vi "SR Volume.vi"() -> ()   [LabVIEW 2012]
uses:
  user.lib/SpectralRadar.llb/Data.lvclass
  user.lib/SpectralRadar.llb/Coloring.lvclass
  user.lib/SpectralRadar.llb/Colored Data.lvclass
  user.lib/SpectralRadar.llb/Colorscheme Selection.ctl
  <vilib>/Math Plots/3D Math Plots/3D Surface/3D Surface XCtrl/3D Surface.xctl
  <vilib>/Utility/error.llb/DialogType.ctl
  user.lib/SpectralRadar.llb/Coloring Byteorder.ctl
  user.lib/SpectralRadar.llb/Probe Parameter Int Selection.ctl
  user.lib/SpectralRadar.llb/Processing Parameter Int Selection.ctl
  user.lib/SpectralRadar.llb/Data Export Format Selection.ctl
  user.lib/SpectralRadar.llb/Colored Data Export Format Selection.ctl
  user.lib/SpectralRadar.llb/Normal Direction Selection.ctl
  user.lib/SpectralRadar.llb/Calibration Selection.ctl
  user.lib/SpectralRadar.llb/display Data 2D as Surface.vi
  user.lib/SpectralRadar.llb/set Scan Output.vi
  user.lib/SpectralRadar.llb/display Data 2D.vi
  user.lib/SpectralRadar.llb/OCT Device.lvclass
  user.lib/SpectralRadar.llb/LabVIEW Helper.lvlib
  user.lib/SpectralRadar.llb/Processing.lvclass
  user.lib/SpectralRadar.llb/Probe.lvclass
  user.lib/SpectralRadar.llb/Scan Pattern.lvclass
  user.lib/SpectralRadar.llb/Settings.lvclass
  user.lib/SpectralRadar.llb/Raw Data.lvclass
  user.lib/SpectralRadar.llb/Post Processing.lvlib
  user.lib/SpectralRadar.llb/ImageField.lvclass
  user.lib/SpectralRadar.llb/FullRange.lvclass
  user.lib/SpectralRadar.llb/FileSelection.lvlib
panel:
  in  "Opacity":sgl(slide) scale=0.0..1.0
  in  "Shift Y [mm]":dbl
  in  "Shift X [mm]":dbl
  out "Filtered Surface":refnum<class "Data.lvclass">
  in  "Color Scheme":T1
  in  "Options":bool
  out "Colored Data":refnum<class "Colored Data.lvclass">
  out "Coloring":refnum<class "Coloring.lvclass">
  out "Surface":refnum<class "Data.lvclass">
  out "Volume":refnum<class "Data.lvclass">
  in  "Angle [rad]":dbl
  in  "Averaging-Binning-Ratio":dbl(slide) caption="Averaging vs. Binning" min=0.0 max=1.0 step=1.0
  in  "Averaging*Binning":i32(slide)=1 caption="Quality" min=1 max=200 step=1 scale=1.0..200.0
  out "AutoSafe":bool
  out "Progress":i32(slide) max=20 scale=0.0..128.0
  in  "Tab Control":enum32{"B-Scan", "Surface"}(tab)
  in  "Boundries":cluster{sgl, sgl}(slide)={72.22738, 40.64965} scale=-20.0..150.0
  out "Frame":sgl[][](graph)
  in  "X":dbl(slide) max=2.0 scale=0.0..2.0
  in  "Y":dbl(slide) max=3.0 scale=0.0..2.0
  in  "Z":dbl(slide) max=1.600000023841858 scale=0.0..5.12 scale format="%#_2g"
  in  "Level Surface":bool
  in  "Petzval Filter":bool
  in  "Median Filter":bool
  in  "SizeFilter":i32=3 min=3 max=15 step=2
  out "3D Surface":refnum<class "3D Plot Datatype.lvclass">[](xcontrol)
  in  "Export Format":T2(ring)
  out "Image":T3(plugin-control)
  out "Reference Intensity":sgl(slide) min=0 max=1 scale=0.0..1.0
  in  "OnlineDisplay":bool
  in  "Brightness":sgl(slide)=0.49673203 caption="Sharpness" min=0 max=1 scale=0.0..1.0
  in  "Contrast":sgl(slide)=0.53594774 caption="Sharpness" min=0 max=1 scale=0.0..1.0
  in  "Saturation":sgl(slide)=0.5294118 caption="Sharpness" min=0 max=1 scale=0.0..1.0
  in  "Light":i32(slide) min=0 max=100 step=1 scale=0.0..100.0
  in  "Description":string
  in  "Test Mode":bool
  out "Test Mode Indicator":bool
  in  "Window":T4(ring)
  out "FrameRate":sgl format="%#_3g"
  out "SpacingZ":dbl
  in  "Range Y [mm]":dbl=3.5999999046325684 caption="Bereich [mm]" min=0.0 max=10.0 step=0.05000000074505806 format="%_3f"
  out "Spacing Y [µm]":dbl=40.0 min=1.0 max=500.0 step=1.0 format="%#_3g"
  in  "Number Scans Y":i32=50 min=10 max=1000 step=1
  in  "Save":bool
  in  "Recalibrate":bool
  in  "Range X [mm]":dbl=2.5999999046325684 caption="Bereich [mm]" min=0.05000000074505806 max=10.0 step=0.05000000074505806 format="%_3f"
  out "Spacing X [µm]":dbl=2.0 min=1.0 max=500.0 step=1.0 format="%#_3g"
  in  "Number Scans X":i32=500 min=100 max=2000 step=1
  in  "Measure":bool
  in  "QuitApp":bool
  # "Stability"
  # "SNR"
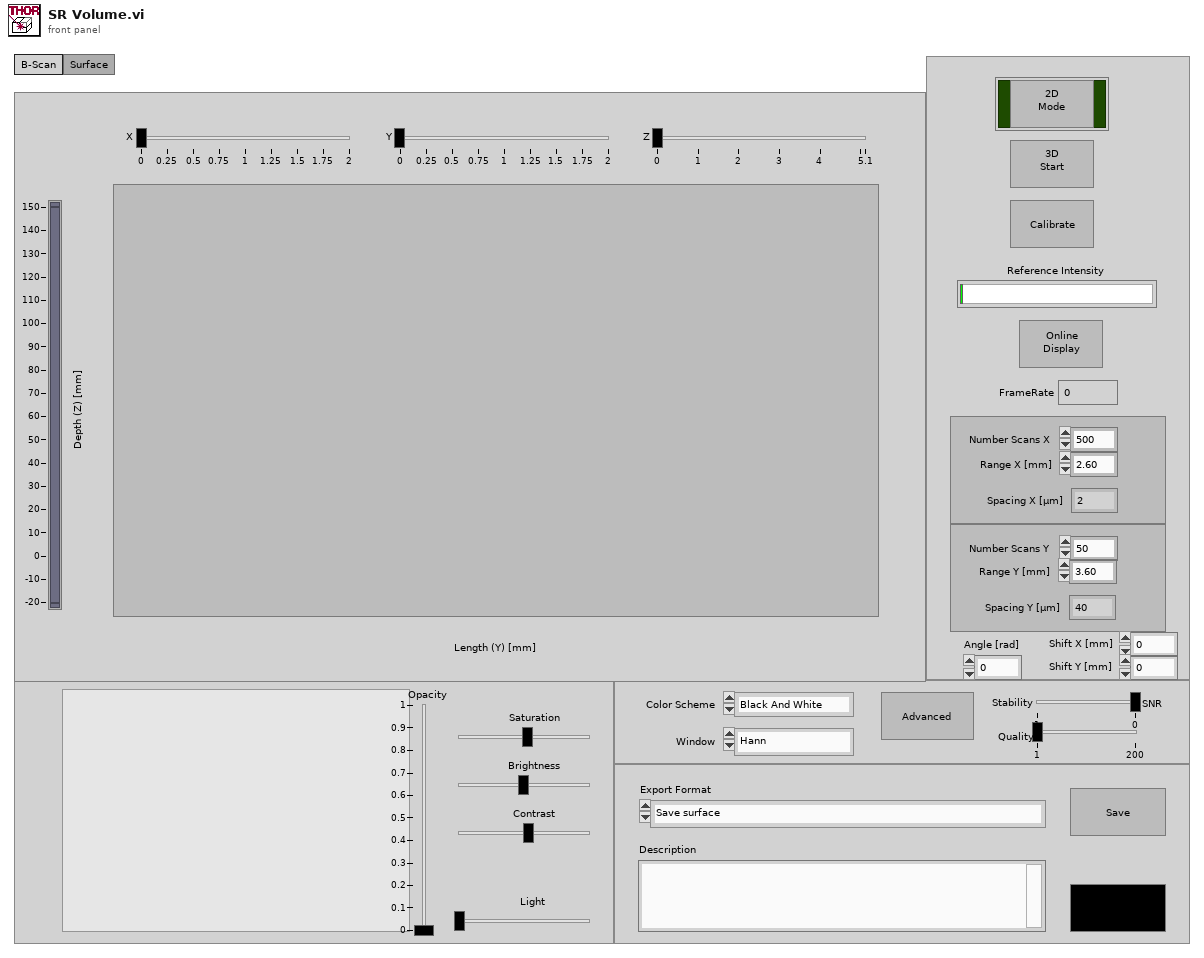
[diagram p1: front panel]
types:
  T1 = typedef "Coloring.lvclass/Colorscheme Selection.ctl" = enum16{"Black And White", "Inverted Black And White", "Color", "Black and Orange", "Black and Red", "Doppler Phase Coloring"}
  T2 = enum16{"Save surface", "Save filtered surface", "Framewise as BMP (*.bmp)", "Framewise as JPG (*.jpg)", "Framewise as PNG (*.png)", "Raw binary floating point (*.raw)", "VFF (*.vff)", "VTK (*.vtk)", "Flexible Image Transport System (*.fits)"}
  T3 = typedef "IMAQ Image.ctl" = refnum<image>
  T4 = enum16{"Hann", "Hamming", "Gauss", "Tapered Cosine", "Blackman", "4 Term B-Harris"}
  T5 = typedef "Coloring.lvclass/Coloring Byteorder.ctl" = enum16{"RGBA32", "BGRA32", "ARGB32", ""}
  T6 = enum16{"Full Well Capacity", "z Spacing", "z Range", "Dynamc Range Min [dB]", "Dynamic Range Low [dB]", "Dynamic Range High [dB]", "Dynamic Range Max [dB]"}
  T7 = typedef "Processing.lvclass/Processing Parameter Int Selection.ctl" = enum32{"Spectrum Averaging", "A-Scan Averaging", "B-Scan Averaging", "Zero Padding", "Number of Threads", "Fourier Averaging"}
  T8 = typedef "Probe.lvclass/Probe Parameter Int Selection.ctl" = enum16{"Apodization Cycles", "Oversampling", "Oversampling Slow Axis", "Speckle Reduction"}
  T9 = typedef "Data.lvclass/Data Export Format Selection.ctl" = enum16{"SRM (Spectral Radar Metafile)", "RAW", "CSV", "TXT", "Table TXT", "Fits", "VFF", "VTK", "TIFF"}
  T10 = typedef "Colored Data.lvclass/Colored Data Export Format Selection.ctl" = enum16{"SRM (Spectral Radar Metafile)", "RAW", "BMP", "PNG", "JPG", "PDF", "TIFF"}
  T11 = enum16{"Asynchronous Continuous", "Asynchronous Finite", "Synchronous"}
  T12 = typedef "Data.lvclass/Normal Direction Selection.ctl" = enum16{"Direction 1", "Direction 2", "Direction 3"}
  T13 = enum8{"Enabled", "Disabled", "Disabled and Grayed Out"}
  T14 = typedef "Processing.lvclass/Calibration Selection.ctl" = enum16{"Offset Errors", "Apodization Spectrum", "Apodization Vector", "Dispersion", "Chirp", "Extended Adjust", "Fixed Pattern"}
  T15 = typedef "DialogType.ctl" = u16
  T16 = typedef "Image Type" = u32
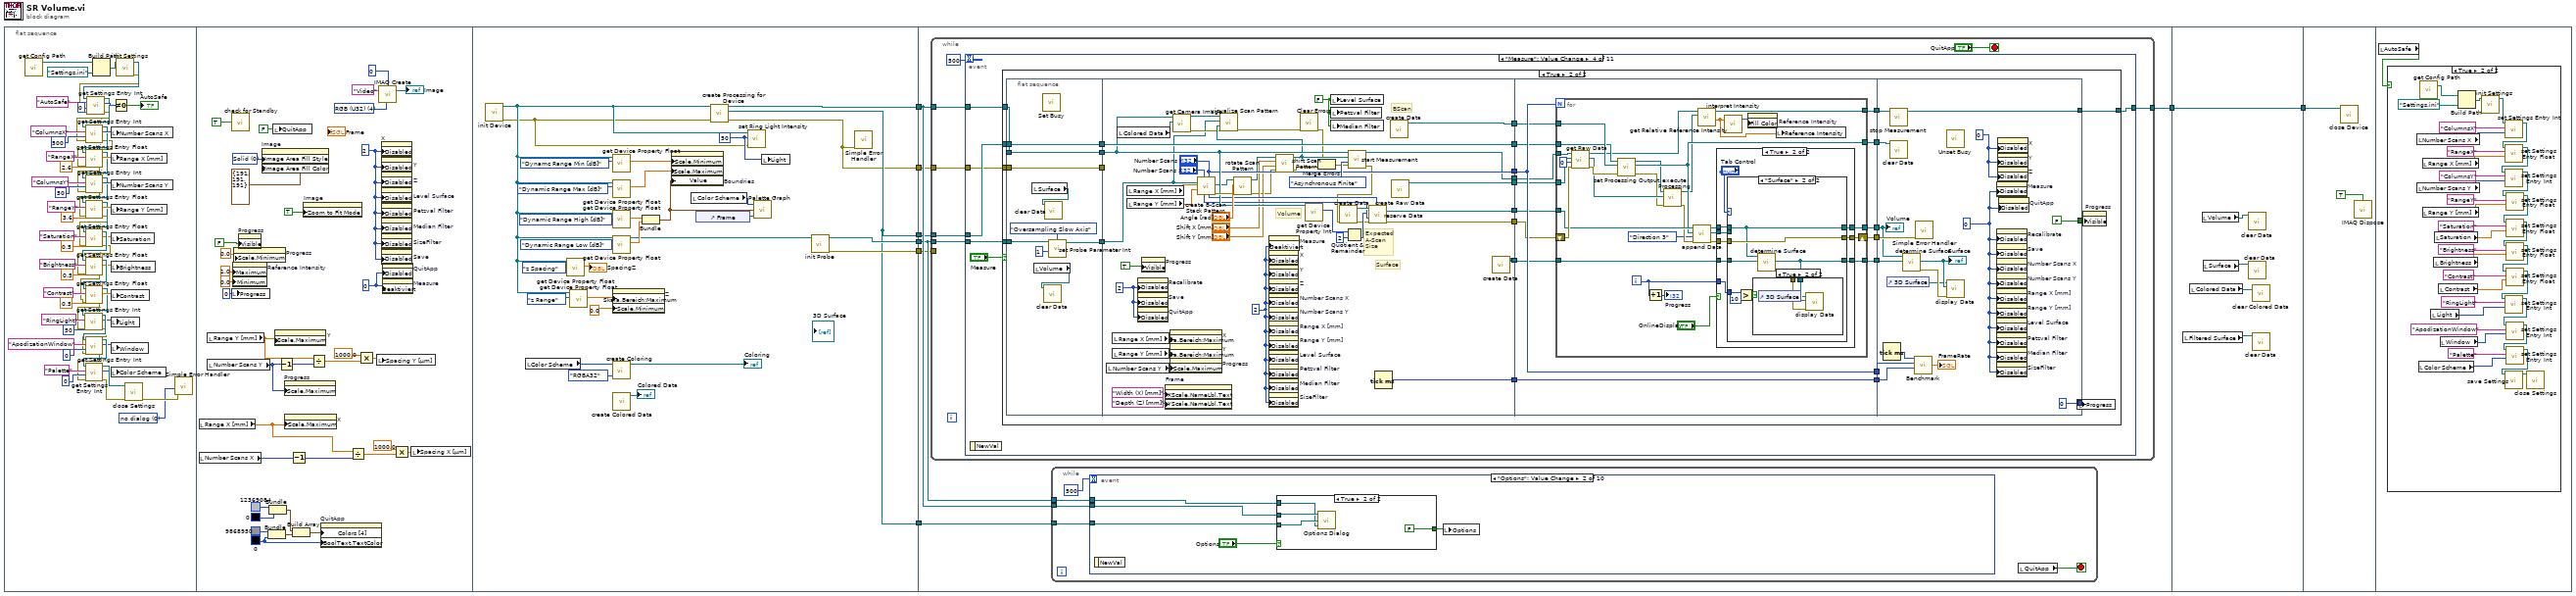
[diagram p0: block diagram]
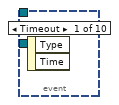
[diagram p2: hidden frame]
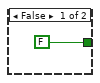
[diagram p3: hidden frame]
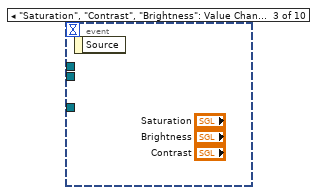
[diagram p4: hidden frame]
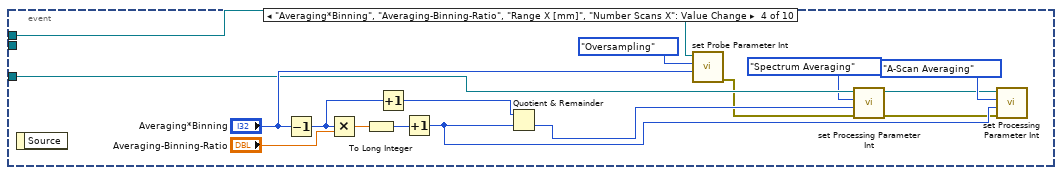
[diagram p5: hidden frame]
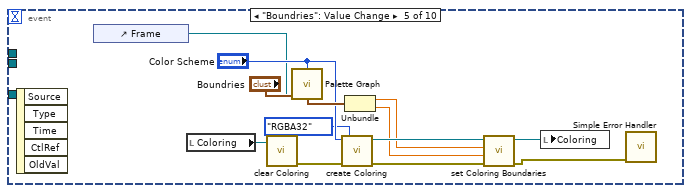
[diagram p6: hidden frame]
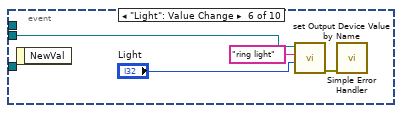
[diagram p7: hidden frame]
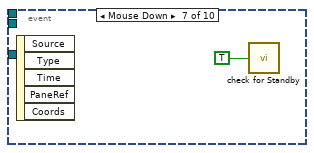
[diagram p8: hidden frame]
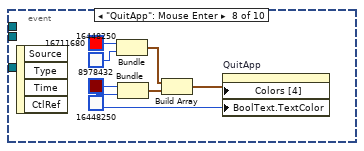
[diagram p9: hidden frame]
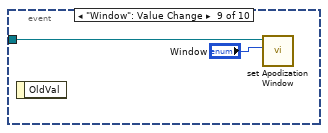
[diagram p10: hidden frame]
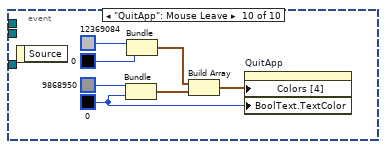
[diagram p11: hidden frame]
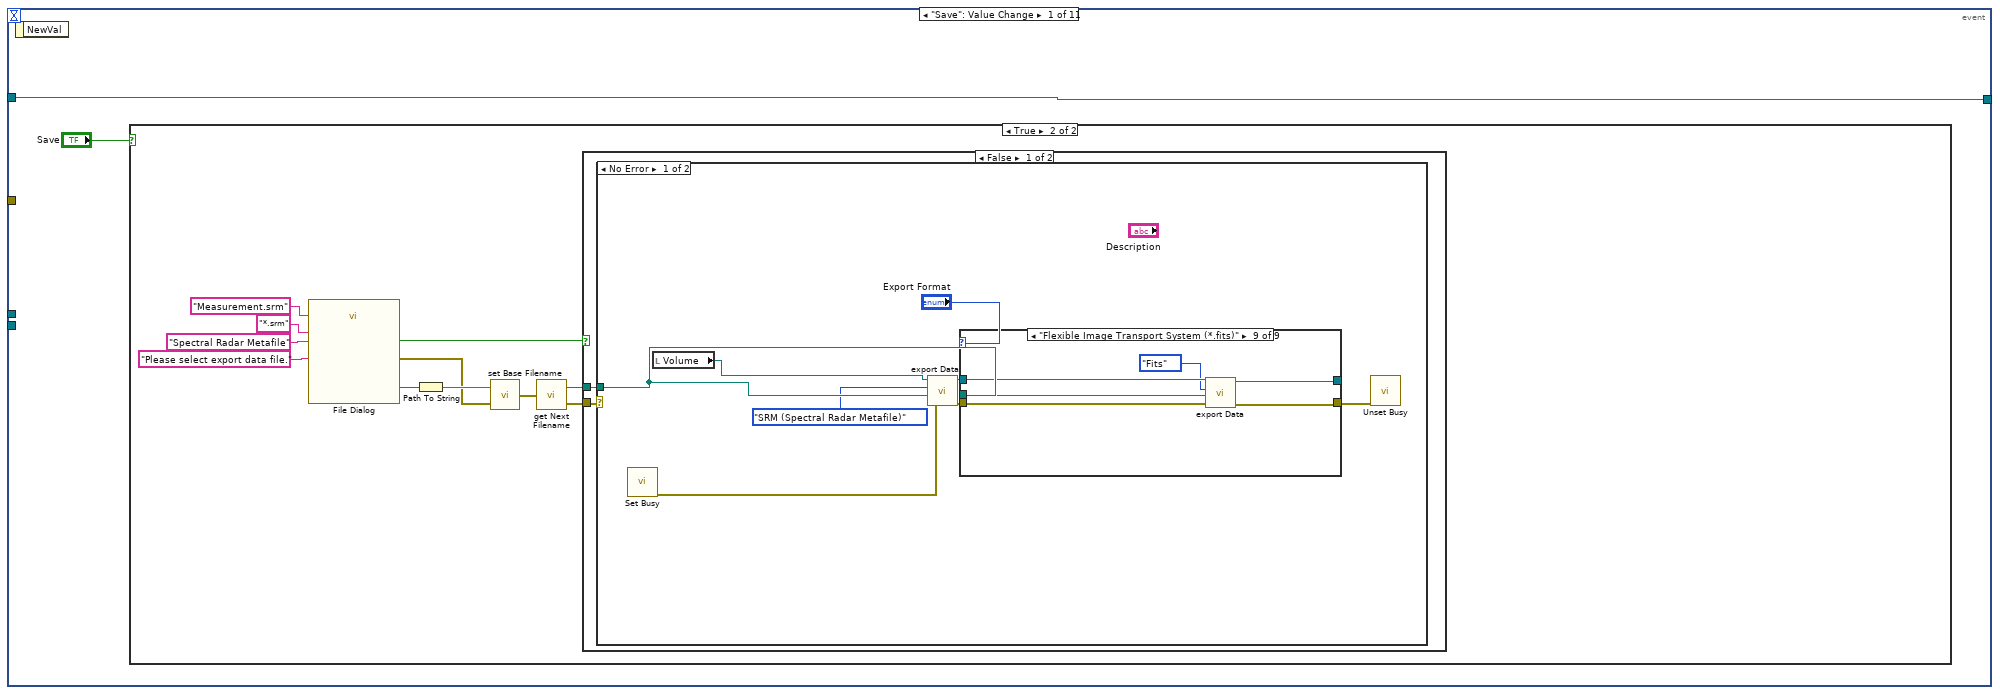
[diagram p12: hidden frame]
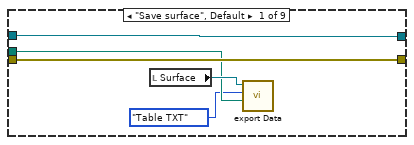
[diagram p14: hidden frame]
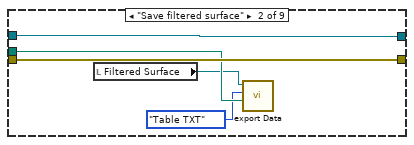
[diagram p15: hidden frame]
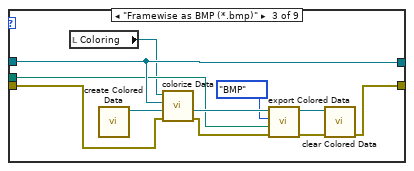
[diagram p16: hidden frame]
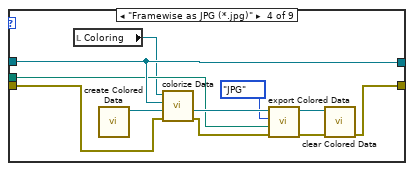
[diagram p17: hidden frame]
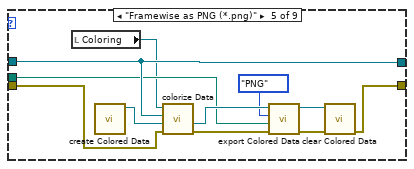
[diagram p18: hidden frame]
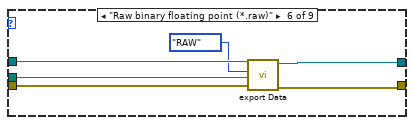
[diagram p19: hidden frame]
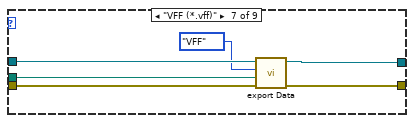
[diagram p20: hidden frame]
diagram:
  n1 = flat-sequence {
    tunnel: [w118] -> w8
    tunnel: [w119] -> w5
    tunnel: [w132] -> w4
    tunnel: [w119] -> w3
    tunnel: [w117] -> w2
    tunnel: [w130] -> w1
    tunnel: w8 -> [w141]
    tunnel: [w142] -> w6
    tunnel: w5 -> [w140]
    tunnel: w4 -> [w138]
    tunnel: w3 -> [w139]
    tunnel: w2 -> [w137]
    tunnel: w1 -> [w136]
    tunnel: [w719] -> w7
    tunnel: w6 -> [w719]
    tunnel: w7 -> [w721]
    frame #0 {
      w12 = T15 0 items=["no dialog", "OK message", "continue or stop message", "OK message + warnings", "continue/stop + warnings"] ("type of dialog (OK msg:1)")
      n2 = call "get Config Path.vi"() -> ("Path"=w22:path)  [unwired: 1 in, 1 out]
      n3 = Build Path(base path=w22, name or relative path=path "Settings.ini" ("Relative \"SpectralRadar.ini\" Path")) -> (appended path=w62:path)
      n4 = call "init Settings.vi"("Path to settings file"=w62) -> ("error out"=w9:errorcluster, "Settings"=w32:refnum<class "Settings.lvclass">)  [unwired: 5 in]
      n5 = call "get Settings Entry Int.vi"("error in (no error)"=w9, "Default Value"=0, "Node Name"="AutoSafe", "Settings"=w32) -> ("error out"=w25:errorcluster, "Value"=w35:i32, "Settings"=w31:refnum<class "Settings.lvclass">)  [unwired: 1 in]
      n6 = call "get Settings Entry Int.vi"("error in (no error)"=w25, "Default Value"=500, "Node Name"="ColumnsX", "Settings"=w31) -> ("error out"=w24:errorcluster, "Value"=w61:i32, "Settings"=w47:refnum<class "Settings.lvclass">)  [unwired: 1 in]
      n7 = call "get Settings Entry Float.vi"("error in (no error)"=w24, "Default Value"=2.6, "Node Name"="RangeX", "Settings"=w47) -> ("error out"=w23:errorcluster, "Value"=w60:dbl, "Settings"=w46:refnum<class "Settings.lvclass">)  [unwired: 1 in]
      n8 = call "get Settings Entry Int.vi"("error in (no error)"=w23, "Default Value"=50, "Node Name"="ColumnsY", "Settings"=w46) -> ("error out"=w21:errorcluster, "Value"=w59:i32, "Settings"=w45:refnum<class "Settings.lvclass">)  [unwired: 1 in]
      n9 = call "get Settings Entry Float.vi"("error in (no error)"=w21, "Default Value"=3.6, "Node Name"="RangeY", "Settings"=w45) -> ("error out"=w20:errorcluster, "Value"=w58:dbl, "Settings"=w44:refnum<class "Settings.lvclass">)  [unwired: 1 in]
      n10 = call "get Settings Entry Float.vi"("error in (no error)"=w20, "Default Value"=0.5, "Node Name"="Saturation", "Settings"=w44) -> ("error out"=w19:errorcluster, "Value"=w37:dbl, "Settings"=w43:refnum<class "Settings.lvclass">)  [unwired: 1 in]
      n11 = call "get Settings Entry Float.vi"("error in (no error)"=w19, "Default Value"=0.5, "Node Name"="Brightness", "Settings"=w43) -> ("error out"=w18:errorcluster, "Value"=w38:dbl, "Settings"=w42:refnum<class "Settings.lvclass">)  [unwired: 1 in]
      n12 = call "get Settings Entry Float.vi"("error in (no error)"=w18, "Default Value"=0.5, "Node Name"="Contrast", "Settings"=w42) -> ("error out"=w17:errorcluster, "Value"=w39:dbl, "Settings"=w30:refnum<class "Settings.lvclass">)  [unwired: 1 in]
      n13 = call "get Settings Entry Int.vi"("error in (no error)"=w17, "Default Value"=50, "Node Name"="RingLight", "Settings"=w30) -> ("error out"=w16:errorcluster, "Value"=w26:i32, "Settings"=w28:refnum<class "Settings.lvclass">)  [unwired: 1 in]
      n14 = call "get Settings Entry Int.vi"("error in (no error)"=w16, "Default Value"=0, "Node Name"="ApodizationWindow", "Settings"=w28) -> ("error out"=w15:errorcluster, "Value"=w40:i32, "Settings"=w41:refnum<class "Settings.lvclass">)  [unwired: 1 in]
      n15 = call "get Settings Entry Int.vi"("error in (no error)"=w15, "Default Value"=0, "Node Name"="Palette", "Settings"=w41) -> ("error out"=w14:errorcluster, "Value"=w11:i32, "Settings"=w36:refnum<class "Settings.lvclass">)  [unwired: 1 in]
      n16 = local write "Number Scans X"(w61) -> ()
      n17 = local write "Range X [mm]"(w60) -> ()
      n18 = local write "Number Scans Y"(w59) -> ()
      n19 = local write "Range Y [mm]"(w58) -> ()
      n20 = local write "Saturation"(w37) -> ()
      n21 = local write "Brightness"(w38) -> ()
      n22 = local write "Contrast"(w39) -> ()
      n23 = local write "Light"(w26) -> ()
      n24 = local write "Window"(w40) -> ()
      n25 = local write "Color Scheme"(w11) -> ()
      n26 = Not Equal To 0?(x=w35) -> (x != 0?=→"AutoSafe":bool)
      n27 = call "close Settings.vi"("error in (no error)"=w14, "Settings"=w36) -> ("error out"=w13:errorcluster)  [unwired: 5 in]
      n28 = call <vilib>:"Simple Error Handler.vi"("type of dialog (OK msg:1)"=w12, "error in (no error)"=w13) -> ()  [unwired: 3 in, 5 out]
    }
    frame #1 {
      w73 = T16 4 items=["Grayscale (U8)", "Grayscale (I16)", "Grayscale (SGL)", "Complex (CSG)", "RGB (U32)", "HSL (U32)", "RGB (U64)", "Grayscale (U16)"] ("Image Type")
      w77 = u8 0 ("Deaktiviert")
      w90 = u8 2 ("Disabled")
      w98 = u32 0
      w103 = u32 0 items=["Default"=3, "Solid"=0, "Hatch"=2] ("Image Area:Background:Fill Style")
      n29 = local read "Range X [mm]"() -> (w78:dbl)
      n30 = local read "Number Scans X"() -> (w80:i32)
      n31 = local read "Range Y [mm]"() -> (w85:dbl)
      n32 = local read "Number Scans Y"() -> (w86:i32)
      n33 = call "check for Standby.vi"("ResetTimer"=TRUE) -> ()  [unwired: 2 out]
      n34 = local write "Progress"(0 ("Progress")) -> ()
      n35 = property on="Reference Intensity" class="Slide (strict)"("Maximum"=1.0 ("Data Entry Limits:Maximum"), "Minimum"=0.0 ("Data Entry Limits:Minimum")) -> ()  [unwired: 2 in, 2 out]
      n36 = property on="Progress" class="Slide (strict)"("Scale.Minimum"=0.0 ("Skalieren.Bereich:Minimum")) -> ()  [unwired: 2 in, 2 out]
      n37 = property on="Progress" class="Slide (strict)"("Visible"=FALSE ("Sichtbar")) -> ()  [unwired: 2 in, 2 out]
      n38 = property on="Image" class="ImageControl"("Image Area Fill Style"=w103, "Image Area Fill Color"=cluster{"Red":u8, "Green":u8, "Blue":u8} {"Red"=191, "Green"=191, "Blue"=191} ("Image Area:Background:Fill Color")) -> ()  [unwired: 2 in, 2 out]
      n39 = Bundle(u32 9868950, w98) -> (w96:cluster{u32, u32})  [unwired: 1 in]
      n40 = Bundle(u32 12369084, u32 0) -> (w95:cluster{u32, u32})  [unwired: 1 in]
      n41 = local write "QuitApp"(FALSE ("QuitApp")) -> ()
      n42 = property on="Y" class="Slide (strict)"("Scale.Maximum"=w85) -> ()  [unwired: 2 in, 2 out]
      n43 = Decrement(x=w86) -> (x-1=w84:i32)
      n44 = property on="Progress" class="Slide (strict)"("Scale.Maximum"=w86) -> ()  [unwired: 2 in, 2 out]
      n45 = property on="X" class="Slide (strict)"("Scale.Maximum"=w78) -> ()  [unwired: 2 in, 2 out]
      n46 = Decrement(x=w80) -> (x-1=w79:i32)
      n47 = Build Array(w95, w96) -> (w97:cluster{u32, u32}[])
      n48 = property on="Image" class="ImageControl"("Zoom to Fit Mode"=TRUE) -> ()  [unwired: 2 in, 2 out]
      n49 = Divide(x=w85, y=w84) -> (x/y=w88:dbl)
      n50 = property on="QuitApp" class="Bool (strict)"("Colors [4]"=w97, "BoolText.TextColor"=w98) -> ()  [unwired: 2 in, 2 out]
      n51 = Divide(x=w78, y=w79) -> (x/y=w82:dbl)
      n52 = Multiply(x=1000.0, y=w88) -> (x*y=w89:dbl)
      n53 = local write "Spacing Y [µm]"(w89) -> ()
      n54 = call "IMAQ Create"("Border Size"=0, "Image Name"="Video", "Image Type"=w73) -> ("New Image"=→"Image":T3)  [unwired: 2 in, 1 out]
      n55 = property on="X" class="Slide (strict)"("Disabled"=w90) -> ()  [unwired: 2 in, 2 out]
      n56 = property on="Y" class="Slide (strict)"("Disabled"=w90) -> ()  [unwired: 2 in, 2 out]
      n57 = property on="Z" class="Slide (strict)"("Disabled"=w90) -> ()  [unwired: 2 in, 2 out]
      n58 = property on="Level Surface" class="Bool (strict)"("Disabled"=w90) -> ()  [unwired: 2 in, 2 out]
      n59 = property on="Petzval Filter" class="Bool (strict)"("Disabled"=w90) -> ()  [unwired: 2 in, 2 out]
      n60 = property on="Median Filter" class="Bool (strict)"("Disabled"=w90) -> ()  [unwired: 2 in, 2 out]
      n61 = property on="SizeFilter" class="DigNum (strict)"("Disabled"=w90) -> ()  [unwired: 2 in, 2 out]
      n62 = property on="Save" class="Bool"("Disabled"=w90) -> ()  [unwired: 2 in, 2 out]
      n63 = property on="QuitApp" class="Bool (strict)"("Disabled"=w77) -> ()  [unwired: 2 in, 2 out]
      n64 = property on="Measure" class="Bool"("Deaktiviert"=w77) -> ()  [unwired: 2 in, 2 out]
      n65 = Multiply(x=sgl 1000.0, y=w82) -> (x*y=w83:dbl)
      n66 = local write "Spacing X [µm]"(w83) -> ()
    }
    frame #2 {
      w135 = 50 ("Intensity[%]")
      n67 = call "init Device.vi"() -> ("error out"=w110:errorcluster, "OCTDevice"=w111:refnum<class "OCT Device.lvclass">)  [unwired: 6 in]
      n68 = local read "Color Scheme"() -> (w108:T1)
      n69 = call "get Device Property Float.vi"("Device Property Float Selection"=T6."z Spacing", "OCTDevice"=w111) -> ("Value"=→"SpacingZ":dbl)  [unwired: 3 in, 2 out]
      n70 = call "get Device Property Float.vi"("Device Property Float Selection"=T6."z Range", "OCTDevice"=w111) -> ("Value"=w115:dbl)  [unwired: 3 in, 2 out]
      n71 = call "get Device Property Float.vi"("Device Property Float Selection"=T6."Dynamc Range Min [dB]", "OCTDevice"=w111) -> ("Value"=w126:dbl)  [unwired: 3 in, 2 out]
      n72 = call "get Device Property Float.vi"("Device Property Float Selection"=T6."Dynamic Range Max [dB]", "OCTDevice"=w111) -> ("Value"=w125:dbl)  [unwired: 3 in, 2 out]
      n73 = call "get Device Property Float.vi"("Device Property Float Selection"=T6."Dynamic Range High [dB]", "OCTDevice"=w111) -> ("Value"=w121:dbl)  [unwired: 3 in, 2 out]
      n74 = call "get Device Property Float.vi"("Device Property Float Selection"=T6."Dynamic Range Low [dB]", "OCTDevice"=w111) -> ("Value"=w120:dbl, "OCTDevice"=w112:refnum<class "OCT Device.lvclass">)  [unwired: 3 in, 1 out]
      n75 = call "create Coloring.vi"("Color Byte Order"=Coloring_Byteorder."RGBA32", "Color Table Selection"=w108) -> ("Coloring"=→"Coloring":refnum<class "Coloring.lvclass">)  [unwired: 4 in, 1 out]
      n76 = property on="Z" class="Slide (strict)"("Skala.Bereich:Maximum"=w115, "Scale.Minimum"=0.0 ("Scale.Range:Minimum")) -> ()  [unwired: 2 in, 2 out]
      n77 = call "create Colored Data.vi"() -> ("Colored Data"=→"Colored Data":refnum<class "Colored Data.lvclass">)  [unwired: 6 in, 1 out]
      n78 = Bundle("Value"=w121, "Value"=w120) -> (w133:cluster{"Value":dbl, "Value":dbl})  [unwired: 1 in]
      n79 = property on="Boundries" class="Slide (strict)"("Scale.Minimum"=w126, "Scale.Maximum"=w125, "Value"=w133) -> ()  [unwired: 2 in, 2 out]
      n80 = local read "Color Scheme"() -> (w109:T1)
      n81 = control-ref of="Frame"() -> (w134:refnum<vi>)
      n82 = call "create Processing for Device.vi"("error in (no error)"=w110, "OCTDevice"=w111) -> ("error out"=w117:errorcluster, "Processing"=w119:refnum<class "Processing.lvclass">, "OCTDevice"=w118:refnum<class "OCT Device.lvclass">)  [unwired: 3 in]
      n83 = call "set Ring Light Intensity.vi"("error in (no error)"=w110, "Intensity[%]"=w135, "OCTDevice"=w111) -> ()  [unwired: 3 in, 2 out]
      n84 = call "Palette Graph.vi"("Reference to the B-scan Graph"=w134, "Boundaries"=w133, "Color Scheme"=w109) -> ()
      n85 = local write "Light"(w135) -> ()
      n86 = call "init Probe.vi"("OCT Device"=w112) -> ("error out"=w130:errorcluster, "GalvoControl"=w132:refnum<class "Probe.lvclass">)  [unwired: 5 in]
      n87 = call <vilib>:"Simple Error Handler.vi"("error in (no error)"=w117) -> ()  [unwired: 4 in, 5 out]
    }
    frame #3 {
      n88 = while {
        tunnel: w141 -> [w210]
        tunnel: [w211] -> w142
        tunnel: w140 -> [w209]
        tunnel: w138 -> [w208]
        tunnel: w137 -> [w207]
        tunnel: w136 -> [_]
        stop <- "QuitApp" stop-if-true
        n89 = event shown="[3] \"Measure\": Value Change" {
          selector: _ -> [_ _ _ _ _ _ _ _ _ _ _]
          dyn-events: _ -> [_ _ _ _ _ _ _ _ _ _ _]
          timeout: 500 -> [_ _ _ _ _ _ _ _ _ _ _]
          tunnel: w210 -> [w215 w322 w358 w366 w542 w653 w664 w670 w686 w701 w714]
          tunnel: [w215 w322 w356 w365 w540 w653 w664 w670 w686 w701 w714] -> w211
          tunnel: w209 -> [_ _ _ w362 w538 _ _ w669 _ _ _]
          tunnel: w208 -> [_ w321 _ w364 w539 _ _ _ _ _ _]
          tunnel: w207 -> [_ _ _ w361 _ _ _ _ _ _ _]
          event "Save": Value Change {
            n90 = event-data() -> ()  [unwired: 1 in, 1 out]
            n91 = case shown="True" "Save" {
              frame False {
              }
              frame True {
                n92 = call "File Dialog"("prompt"="Please select export data file.", "default name"="Measurement.srm", "pattern (all files)"="*.srm", "pattern label"="Spectral Radar Metafile") -> ("selected path"=w220:path, "cancelled"=w218:bool, "error out"=w217:errorcluster)  [unwired: 8 in, 1 out]
                n93 = Path To String(path=w220) -> (string=w219:string)
                n94 = call "set Base Filename.vi"("error in (no error)"=w217, "Base"=w219) -> ("error out"=w226:errorcluster)
                n95 = call "get Next Filename.vi"("error in (no error)"=w226) -> ("Next File Name"=w225:path, "error out"=w216:errorcluster)
                n96 = case shown="False" w218 {
                  tunnel: w225 -> [w228 _]
                  tunnel: w216 -> [w227 _]
                  frame False {
                    n97 = case shown="No Error" w227 {
                      tunnel: w228 -> [w231 _]
                      frame No Error {
                        n98 = call <vilib>:"Set Busy.vi"() -> ("error out"=w233:errorcluster)  [unwired: 10 in, 1 out]
                        n99 = local read "Volume"() -> (w229:refnum<class "Data.lvclass">)
                        n100 = call "export Data.vi"("error in (no error)"=w233, "Export File"=w231, "Data Export Format Selection"=Data_Export_Format_Selection."SRM (Spectral Radar Metafile)" ("Data 2D Export Format Selection"), "Data in"=w229) -> ("error out"=w234:errorcluster, "Data out"=w235:refnum<class "Data.lvclass">)  [unwired: 2 in]
                        n101 = case shown="\"Flexible Image Transport System (*.fits)\"" "Export Format" {
                          tunnel: w235 -> [w240 w245 w257 w268 w279 w285 w291 w296 w303]
                          tunnel: [w240 w245 w257 w268 w279 w284 w290 w297 w302] -> _
                          tunnel: w231 -> [w238 w244 w254 w265 w276 w280 w287 w293 w299]
                          tunnel: w234 -> [w241 w246 w251 w262 w273 w283 w289 w295 w301]
                          tunnel: [w241 w246 w248 w259 w270 w282 w288 w294 w300] -> w232
                          frame "Save surface", Default {
                            n102 = local read "Surface"() -> (w239:refnum<class "Data.lvclass">)
                            n103 = call "export Data.vi"("Export File"=w238, "Data Export Format Selection"=Data_Export_Format_Selection."Table TXT" ("Data 2D Export Format Selection"), "Data in"=w239) -> ()  [unwired: 3 in, 2 out]
                          }
                          frame "Save filtered surface" {
                            n104 = local read "Filtered Surface"() -> (w243:refnum<class "Data.lvclass">)
                            n105 = call "export Data.vi"("Export File"=w244, "Data Export Format Selection"=Data_Export_Format_Selection."Table TXT" ("Data 2D Export Format Selection"), "Data in"=w243) -> ()  [unwired: 3 in, 2 out]
                          }
                          frame "Framewise as BMP (*.bmp)" {
                            n106 = local read "Coloring"() -> (w247:refnum<class "Coloring.lvclass">)
                            n107 = call "create Colored Data.vi"() -> ("Colored Data"=w256:refnum<class "Colored Data.lvclass">)  [unwired: 6 in, 1 out]
                            n108 = call "colorize Data.vi"("error in (no error)"=w251, "Colored Data"=w256, "Data"=w257, "Coloring in"=w247) -> ("error out"=w250:errorcluster, "Colored Data"=w255:refnum<class "Colored Data.lvclass">)  [unwired: 2 out]
                            n109 = call "export Colored Data.vi"("error in (no error)"=w250, "File Name"=w254, "Colored Data Export Format Selection"=Colored_Data_Export_Format_Selection."BMP", "Colored Data in"=w255) -> ("error out"=w249:errorcluster, "Colored Data out"=w252:refnum<class "Colored Data.lvclass">)  [unwired: 2 in]
                            n110 = call "clear Colored Data.vi"("error in (no error)"=w249, "Colored Data"=w252) -> ("error out"=w248:errorcluster)  [unwired: 5 in]
                          }
                          frame "Framewise as JPG (*.jpg)" {
                            n111 = local read "Coloring"() -> (w258:refnum<class "Coloring.lvclass">)
                            n112 = call "create Colored Data.vi"() -> ("Colored Data"=w267:refnum<class "Colored Data.lvclass">)  [unwired: 6 in, 1 out]
                            n113 = call "colorize Data.vi"("error in (no error)"=w262, "Colored Data"=w267, "Data"=w268, "Coloring in"=w258) -> ("error out"=w261:errorcluster, "Colored Data"=w266:refnum<class "Colored Data.lvclass">)  [unwired: 2 out]
                            n114 = call "export Colored Data.vi"("error in (no error)"=w261, "File Name"=w265, "Colored Data Export Format Selection"=Colored_Data_Export_Format_Selection."JPG", "Colored Data in"=w266) -> ("error out"=w260:errorcluster, "Colored Data out"=w263:refnum<class "Colored Data.lvclass">)  [unwired: 2 in]
                            n115 = call "clear Colored Data.vi"("error in (no error)"=w260, "Colored Data"=w263) -> ("error out"=w259:errorcluster)  [unwired: 5 in]
                          }
                          frame "Framewise as PNG (*.png)" {
                            n116 = local read "Coloring"() -> (w269:refnum<class "Coloring.lvclass">)
                            n117 = call "create Colored Data.vi"() -> ("Colored Data"=w278:refnum<class "Colored Data.lvclass">)  [unwired: 6 in, 1 out]
                            n118 = call "colorize Data.vi"("error in (no error)"=w273, "Colored Data"=w278, "Data"=w279, "Coloring in"=w269) -> ("error out"=w272:errorcluster, "Colored Data"=w277:refnum<class "Colored Data.lvclass">)  [unwired: 2 out]
                            n119 = call "export Colored Data.vi"("error in (no error)"=w272, "File Name"=w276, "Colored Data Export Format Selection"=Colored_Data_Export_Format_Selection."PNG", "Colored Data in"=w277) -> ("error out"=w271:errorcluster, "Colored Data out"=w274:refnum<class "Colored Data.lvclass">)  [unwired: 2 in]
                            n120 = call "clear Colored Data.vi"("error in (no error)"=w271, "Colored Data"=w274) -> ("error out"=w270:errorcluster)  [unwired: 5 in]
                          }
                          frame "Raw binary floating point (*.raw)" {
                            n121 = call "export Data.vi"("error in (no error)"=w283, "Export File"=w280, "Data Export Format Selection"=Data_Export_Format_Selection."RAW" ("Data 2D Export Format Selection"), "Data in"=w285) -> ("error out"=w282:errorcluster, "Data out"=w284:refnum<class "Data.lvclass">)  [unwired: 2 in]
                          }
                          frame "VFF (*.vff)" {
                            n122 = call "export Data.vi"("error in (no error)"=w289, "Export File"=w287, "Data Export Format Selection"=Data_Export_Format_Selection."VFF" ("Data 2D Export Format Selection"), "Data in"=w291) -> ("error out"=w288:errorcluster, "Data out"=w290:refnum<class "Data.lvclass">)  [unwired: 2 in]
                          }
                          frame "VTK (*.vtk)" {
                            n123 = call "export Data.vi"("error in (no error)"=w295, "Export File"=w293, "Data Export Format Selection"=Data_Export_Format_Selection."VTK" ("Data 2D Export Format Selection"), "Data in"=w296) -> ("error out"=w294:errorcluster, "Data out"=w297:refnum<class "Data.lvclass">)  [unwired: 2 in]
                          }
                          frame "Flexible Image Transport System (*.fits)" {
                            n124 = call "export Data.vi"("error in (no error)"=w301, "Export File"=w299, "Data Export Format Selection"=Data_Export_Format_Selection."Fits" ("Data 2D Export Format Selection"), "Data in"=w303) -> ("error out"=w300:errorcluster, "Data out"=w302:refnum<class "Data.lvclass">)  [unwired: 2 in]
                          }
                        }
                        n125 = call <vilib>:"Unset Busy.vi"("error in (no error)"=w232) -> ()  [unwired: 10 in, 1 out]
                      }
                      frame Error {
                      }
                    }
                  }
                  frame True {
                  }
                }
              }
            }
          }
          event "Median Filter", "Level Surface", "Petzval Filter", "SizeFilter", "Spacing Y [µm]", "Spacing X [µm]": Value Change {
            n126 = event-data() -> ()  [unwired: 1 in, 1 out]
            n127 = local read "Filtered Surface"() -> (w305:refnum<class "Data.lvclass">)
            n128 = call "clear Data.vi"("Data"=w305) -> ("error out"=w306:errorcluster)  [unwired: 6 in]
            n129 = local read "Surface"() -> (w317:refnum<class "Data.lvclass">)
            n130 = call "create Data.vi"("error in (no error)"=w306) -> ("Data"=w316:refnum<class "Data.lvclass">)  [unwired: 5 in, 1 out]
            n131 = call "copy Data.vi"("Data Destination in"=w316, "Data Source in"=w317) -> ("error out"=w313:errorcluster, "Data Destination out"=w315:refnum<class "Data.lvclass">)  [unwired: 3 in, 1 out]
            n132 = case shown="True" "Median Filter" {
              tunnel: w313 -> [w344 w347]
              tunnel: w315 -> [w345 w349]
              tunnel: [w345 w348] -> w314
              tunnel: [w344 w346] -> w312
              frame False {
              }
              frame True {
                n133 = call "median Filter.vi"("error in (no error)"=w347, "Rank"="SizeFilter", "Data in"=w349) -> ("error out"=w346:errorcluster, "Data out"=w348:refnum<class "Data.lvclass">)  [unwired: 3 in]
              }
            }
            n134 = case shown="True" "Petzval Filter" {
              tunnel: w321 -> [_ _]
              tunnel: w314 -> [w330 w336]
              tunnel: w312 -> [w329 w343]
              tunnel: [w330 w335] -> w311
              tunnel: [w329 w332] -> w310
              frame False {
              }
              frame True {
                n135 = call "get Config Path.vi"() -> ("Path"=w340:path)  [unwired: 1 in, 1 out]
                n136 = call "create Image Field.vi"("error in (no error)"=w343) -> ("error out"=w341:errorcluster, "ImageField out"=w342:refnum<class "ImageField.lvclass">)  [unwired: 5 in]
                n137 = Build Path(base path=w340, name or relative path=path "ImageField.dat") -> (appended path=w337:path)
                n138 = call "load Image Field.vi"("error in (no error)"=w341, "Path"=w337, "ImageField in"=w342) -> ("error out"=w338:errorcluster, "ImageField out"=w339:refnum<class "ImageField.lvclass">)  [unwired: 3 in]
                n139 = call "correct Surface.vi"("error in (no error)"=w338, "Surface Data in"=w336, "ImageField in"=w339) -> ("error out"=w333:errorcluster, "Surface Data out"=w335:refnum<class "Data.lvclass">, "ImageField out"=w334:refnum<class "ImageField.lvclass">)  [unwired: 2 in]
                n140 = call "clear Image Field.vi"("error in (no error)"=w333, "ImageField in"=w334) -> ("error out"=w332:errorcluster)  [unwired: 5 in]
              }
            }
            n141 = case shown="True" "Level Surface" {
              tunnel: [w324 w327] -> w308
              tunnel: [w323 w328] -> w309
              tunnel: w311 -> [w324 w326]
              tunnel: w310 -> [w323 w325]
              frame False {
              }
              frame True {
                n142 = call "level Data.vi"("error in (no error)"=w325, "Data in"=w326) -> ("error out"=w328:errorcluster, "Data out"=w327:refnum<class "Data.lvclass">)  [unwired: 4 in]
              }
            }
            n143 = control-ref of="3D Surface"() -> (w304:refnum<vi>)
            n144 = call-poly "display Data.vi"("error in (no error)"=w309, "Data in"=w308, "3D Surface Refnum"=w304) -> ("Data out"=→"Filtered Surface":refnum<class "Data.lvclass">)  [unwired: 2 in, 2 out]
          }
          event Timeout {
            n145 = event-data() -> ()  [unwired: 1 in, 1 out]
            n146 = call "check for Standby.vi"() -> ("TimeOut"=w360:bool)  [unwired: 1 in, 1 out]
            n147 = call "activate Standby.vi"("StandBy"=w360, "OCTDevice"=w358) -> ("OCTDevice"=w357:refnum<class "OCT Device.lvclass">)  [unwired: 4 in, 1 out]
            n148 = local read "Colored Data"() -> (w359:refnum<class "Colored Data.lvclass">)
            n149 = call "get Camera Image.vi"("Colored Data in"=w359, "OCTDevice in"=w357) -> ("error out"=w353:errorcluster, "Colored Data out"=w354:refnum<class "Colored Data.lvclass">, "OCTDevice out"=w356:refnum<class "OCT Device.lvclass">)  [unwired: 5 in]
            n150 = local read "Image"() -> (w355:T3)
            n151 = call "update Colored Data IMAQ Image.vi"("error in (no error)"=w353, "Image in"=w355, "Colored Data"=w354) -> ("error out"=w351:errorcluster, "Image out"=w352:T3)  [unwired: 2 in, 1 out]
            n152 = local write "Image"(w352) -> ()
            n153 = call <vilib>:"Clear Errors.vi"("error in (no error)"=w351) -> ()  [unwired: 6 in, 1 out]
          }
          event "Measure": Value Change {
            n154 = event-data() -> ()  [unwired: 1 in, 1 out]
            n155 = case shown="True" "Measure" {
              tunnel: w366 -> [w367 w390]
              tunnel: [w367 w394] -> w365
              tunnel: w364 -> [_ w393]
              tunnel: w362 -> [_ w392]
              tunnel: w361 -> [_ w391]
              frame False {
              }
              frame True {
                n156 = flat-sequence {
                  tunnel: w391 -> [w401]
                  tunnel: w392 -> [w402]
                  tunnel: w393 -> [w398]
                  tunnel: w390 -> [w403]
                  tunnel: [w403] -> w389
                  tunnel: [w397] -> w388
                  tunnel: [w402] -> w387
                  tunnel: [w401] -> w386
                  tunnel: ["Number Scans Y"] -> w385
                  tunnel: [w441] -> w384
                  tunnel: [w415] -> w383
                  tunnel: [w433] -> w382
                  tunnel: [w432] -> w381
                  tunnel: [w431] -> w380
                  tunnel: [w427] -> w379
                  tunnel: [w430] -> w378
                  tunnel: w389 -> [w425]
                  tunnel: w388 -> [w404]
                  tunnel: w387 -> [w433]
                  tunnel: w386 -> [_]
                  tunnel: [w408] -> w368
                  tunnel: [w462] -> w377
                  tunnel: w385 -> [w462]
                  tunnel: [w461] -> w376
                  tunnel: [w460] -> w375
                  tunnel: w384 -> [w460]
                  tunnel: w383 -> [w458]
                  tunnel: w382 -> [w457]
                  tunnel: w381 -> [w459]
                  tunnel: w380 -> [w456]
                  tunnel: w379 -> [w455]
                  tunnel: [w454] -> w374
                  tunnel: [w453] -> w373
                  tunnel: [w452] -> w372
                  tunnel: w378 -> [w451]
                  tunnel: [w450] -> w371
                  tunnel: w368 -> [w449]
                  tunnel: w377 -> [w536]
                  tunnel: [0 ("Progress")] -> w370
                  tunnel: [FALSE ("Sichtbar")] -> w369
                  tunnel: w376 -> [w533]
                  tunnel: [w532] -> w394
                  tunnel: w375 -> [w531]
                  tunnel: w374 -> [w528]
                  tunnel: w373 -> [w527]
                  tunnel: w372 -> [w524]
                  tunnel: w371 -> [w525]
                  frame #0 {
                    n157 = local read "Surface"() -> (w400:refnum<class "Data.lvclass">)
                    n158 = local read "Volume"() -> (w399:refnum<class "Data.lvclass">)
                    n159 = call <vilib>:"Set Busy.vi"() -> ()  [unwired: 10 in, 2 out]
                    n160 = call "clear Data.vi"("Data"=w399) -> ()  [unwired: 6 in, 1 out]
                    n161 = call "clear Data.vi"("Data"=w400) -> ()  [unwired: 6 in, 1 out]
                    n162 = call "set Probe Parameter Int.vi"("Value"=1, "Probe Parameter Int"=Probe_Parameter_Int_Selection."Oversampling Slow Axis", "GalvoControl"=w398) -> ("GalvoControl"=w397:refnum<class "Probe.lvclass">)  [unwired: 3 in, 1 out]
                  }
                  frame #1 {
                    w439 = FALSE ("Level Surface")
                    w442 = u8 2 ("Deaktiviert")
                    w440 = u8 2
                    # "Expected\nA-Scan\nSize"
                    # "Surface"
                    # "Volume"
                    # "BScan"
                    n163 = local read "Number Scans Y"() -> (w447:i32)
                    n164 = local read "Range X [mm]"() -> (w446:dbl)
                    n165 = local read "Range Y [mm]"() -> (w448:dbl)
                    n166 = local read "Colored Data"() -> (w429:refnum<class "Colored Data.lvclass">)
                    n167 = local read "Range X [mm]"() -> (w438:dbl)
                    n168 = local read "Range Y [mm]"() -> (w437:dbl)
                    n169 = property on="Recalibrate" class="Bool"("Disabled"=w442) -> ()  [unwired: 2 in, 2 out]
                    n170 = property on="Save" class="Bool"("Disabled"=w442) -> ()  [unwired: 2 in, 2 out]
                    n171 = property on="QuitApp" class="Bool (strict)"("Disabled"=w442) -> ()  [unwired: 2 in, 2 out]
                    n172 = property on="Progress" class="Slide (strict)"("Visible"=TRUE ("Sichtbar")) -> ()  [unwired: 2 in, 2 out]
                    n173 = property on="Frame" class="IntGraph (strict)"("XScale.NameLbl.Text"="Width (X) [mm]" ("X Scale.Name Label.Text"), "YScale.NameLbl.Text"="Depth (Z) [mm]" ("Y Scale.Name Label.Text")) -> ()  [unwired: 2 in, 2 out]
                    n174 = property on="X" class="Slide (strict)"("Skala.Bereich:Maximum"=w446) -> ()  [unwired: 2 in, 2 out]
                    n175 = property on="Y" class="Slide (strict)"("Skala.Bereich:Maximum"=w448) -> ()  [unwired: 2 in, 2 out]
                    n176 = property on="Progress" class="Slide (strict)"("Scale.Maximum"=w447) -> ()  [unwired: 2 in, 2 out]
                    n177 = call "get Camera Image.vi"("Colored Data in"=w429, "OCTDevice in"=w425) -> ("error out"=w407:errorcluster, "OCTDevice out"=w405:refnum<class "OCT Device.lvclass">)  [unwired: 5 in, 1 out]
                    n178 = call "create B-Scan Stack Pattern.vi"("Size Y"="Number Scans Y", "Size X"="Number Scans X", "Range Y"=w437, "Range X"=w438, "Probe"=w404) -> ("error out"=w434:errorcluster, "Scan Pattern"=w417:refnum<class "Scan Pattern.lvclass">)  [unwired: 2 in, 1 out]
                    n179 = call "rotate Scan Pattern.vi"("error in (no error)"=w434, "Angle"="Angle [rad]", "ScanPattern"=w417) -> ("error out"=w413:errorcluster, "ScanPattern"=w420:refnum<class "Scan Pattern.lvclass">)  [unwired: 3 in]
                    n180 = property on="X" class="Slide (strict)"("Disabled"=w440) -> ()  [unwired: 2 in, 2 out]
                    n181 = property on="Y" class="Slide (strict)"("Disabled"=w440) -> ()  [unwired: 2 in, 2 out]
                    n182 = property on="Z" class="Slide (strict)"("Disabled"=w440) -> ()  [unwired: 2 in, 2 out]
                    n183 = property on="Number Scans X" class="DigNum (strict)"("Disabled"=w440) -> ()  [unwired: 2 in, 2 out]
                    n184 = property on="Number Scans Y" class="DigNum (strict)"("Disabled"=w440) -> ()  [unwired: 2 in, 2 out]
                    n185 = property on="Range X [mm]" class="DigNum (strict)"("Disabled"=w440) -> ()  [unwired: 2 in, 2 out]
                    n186 = property on="Range Y [mm]" class="DigNum (strict)"("Disabled"=w440) -> ()  [unwired: 2 in, 2 out]
                    n187 = property on="Level Surface" class="Bool (strict)"("Disabled"=w440) -> ()  [unwired: 2 in, 2 out]
                    n188 = property on="Petzval Filter" class="Bool (strict)"("Disabled"=w440) -> ()  [unwired: 2 in, 2 out]
                    n189 = property on="Median Filter" class="Bool (strict)"("Disabled"=w440) -> ()  [unwired: 2 in, 2 out]
                    n190 = property on="SizeFilter" class="DigNum (strict)"("Disabled"=w440) -> ()  [unwired: 2 in, 2 out]
                    n191 = property on="Measure" class="Bool"("Deaktiviert"=w440) -> ()  [unwired: 2 in, 2 out]
                    n192 = call "shift Scan Pattern.vi"("error in (no error)"=w413, "Shift Y"="Shift Y [mm]", "Shift X"="Shift X [mm]", "Scan Pattern in"=w420) -> ("error out"=w412:errorcluster, "Scan Pattern out"=w416:refnum<class "Scan Pattern.lvclass">)  [unwired: 2 in]
                    n193 = call "visualize Scan Pattern.vi"("error in (no error)"=w407, "Scan Pattern in"=w416, "Probe"=w404, "OCT Device"=w405) -> ("error out"=w406:errorcluster)  [unwired: 1 in, 3 out]
                    n194 = call <vilib>:"Clear Errors.vi"("error in (no error)"=w406) -> ("error out"=w410:errorcluster)  [unwired: 6 in]
                    n195 = call "get Device Property Int.vi"("OCTDevice"=w425) -> ("Value"=w426:i32)  [unwired: 4 in, 2 out]
                    n196 = Merge Errors(w410, w412) -> (w411:errorcluster)
                    n197 = local write "Level Surface"(w439) -> ()
                    n198 = local write "Petzval Filter"(w439) -> ()
                    n199 = local write "Median Filter"(w439) -> ()
                    n200 = Quotient & Remainder(x=w426, y=2) -> (floor(x/y)=w421:i32)  [unwired: 1 out]
                    n201 = call "start Measurement.vi"("error in (no error)"=w411, "Acquisition Type"=T11."Asynchronous Finite", "Scan Pattern"=w416, "OCTDevice"=w425) -> ("error out"=w409:errorcluster, "OCTDevice"=w415:refnum<class "OCT Device.lvclass">)  [unwired: 1 in, 1 out]
                    n202 = call "create Data.vi"("error in (no error)"=w409) -> ("error out"=w414:errorcluster, "Data"=w428:refnum<class "Data.lvclass">)  [unwired: 5 in]
                    n203 = call "reserve Data.vi"("Size 3"="Number Scans Y", "error in (no error)"=w414, "Size 2"="Number Scans X", "Size 1"=w421, "Data in"=w428) -> ("error out"=w408:errorcluster, "Data out"=w427:refnum<class "Data.lvclass">)  [unwired: 3 in]
                    n204 = Tick Count (ms)() -> (millisecond timer value=w441:u32)
                    n205 = call "create Data.vi"() -> ("Data"=w432:refnum<class "Data.lvclass">)  [unwired: 6 in, 1 out]
                    n206 = call "create Raw Data.vi"() -> ("Raw Data"=w431:refnum<class "Raw Data.lvclass">)  [unwired: 6 in, 1 out]
                    n207 = call "create Data.vi"() -> ("Data"=w430:refnum<class "Data.lvclass">)  [unwired: 6 in, 1 out]
                  }
                  frame #2 {
                    n208 = for {
                      N: w462 -> [_]
                      tunnel: [w470] -> w461
                      tunnel: w459 -> [w487]
                      tunnel: w458 -> [w488]
                      tunnel: w457 -> [w486]
                      tunnel: w456 -> [w484]
                      tunnel: w455 -> [w479]
                      tunnel: [w478] -> w453
                      tunnel: [w472] -> w452
                      tunnel: w451 -> [w466]
                      tunnel: [w465] -> w450
                      shift-right: [w482] -> w454
                      shift-left: w449 -> [w489]
                      i -> [w490]
                      n209 = call "get Raw Data.vi"("error in (no error)"=w489, "Camera Index"=0, "RawData in"=w484, "OCTDevice in"=w488) -> ("error out"=w485:errorcluster, "RawData out"=w483:refnum<class "Raw Data.lvclass">, "OCTDevice out"=w471:refnum<class "OCT Device.lvclass">)  [unwired: 1 in]
                      n210 = call-poly "set Processing Output.vi"("error in (no error)"=w485, "Data"=w487, "Processing"=w486) -> ("error out"=w480:errorcluster, "Data"=w478:refnum<class "Data.lvclass">, "Processing"=w468:refnum<class "Processing.lvclass">)  [unwired: 2 in]
                      n211 = Increment(x=w490) -> (x+1=→"Progress":i32)
                      n212 = call "execute Processing.vi"("error in (no error)"=w480, "Raw Data"=w483, "Processing"=w468) -> ("error out"=w475:errorcluster, "Processing"=w467:refnum<class "Processing.lvclass">)  [unwired: 2 in, 1 out]
                      n213 = call "append Data.vi"("error in (no error)"=w475, "Normal Direction"=Normal_Direction_Selection."Direction 3", "Data to append in"=w478, "Data in"=w479) -> ("error out"=w476:errorcluster, "Data to append out"=w477:refnum<class "Data.lvclass">, "Data out"=w473:refnum<class "Data.lvclass">)  [unwired: 1 in]
                      n214 = call "get Relative Reference Intensity.vi"("Processing"=w467, "OCTDevice"=w471) -> ("Relative Reference Intensity"=w464:dbl, "OCTDevice"=w470:refnum<class "OCT Device.lvclass">)  [unwired: 2 in, 2 out]
                      n215 = case shown="True" "OnlineDisplay" {
                        tunnel: w490 -> [_ w495]
                        tunnel: w477 -> [_ w502]
                        tunnel: w476 -> [w494 w501]
                        tunnel: [w494 w500] -> w482
                        tunnel: w473 -> [w493 w499]
                        tunnel: [w493 w498] -> w472
                        tunnel: w466 -> [w492 w497]
                        tunnel: [w492 w496] -> w465
                        frame False {
                        }
                        frame True {
                          n216 = case shown="\"Surface\"" "Tab Control" {
                            tunnel: w502 -> [w509 _]
                            tunnel: w501 -> [w507 w517]
                            tunnel: [w506 w517] -> w500
                            tunnel: w499 -> [w505 w516]
                            tunnel: [w505 w516] -> w498
                            tunnel: w497 -> [w504 w515]
                            tunnel: [w504 w514] -> w496
                            tunnel: w495 -> [_ w512]
                            frame "B-Scan", Default {
                              n217 = control-ref of="Frame"() -> (w508:refnum<vi>)
                              n218 = call-poly "display Data.vi"("error in (no error)"=w507, "Data in"=w509, "IntGraph Refnum"=w508) -> ("error out"=w506:errorcluster)  [unwired: 2 in, 2 out]
                            }
                            frame "Surface" {
                              n219 = Greater?(x=w512, y=10) -> (0:w510:bool)
                              n220 = call "determine Surface.vi"("Surface Data in"=w515, "Data in"=w516) -> ("error out"=w513:errorcluster, "Surface Data out"=w514:refnum<class "Data.lvclass">)  [unwired: 3 in, 1 out]
                              n221 = case shown="True" w510 {
                                tunnel: w514 -> [_ w520]
                                tunnel: w513 -> [_ w519]
                                frame False {
                                }
                                frame True {
                                n222 = control-ref of="3D Surface"() -> (w518:refnum<vi>)
                                n223 = call-poly "display Data.vi"("error in (no error)"=w519, "Data in"=w520, "3D Surface Refnum"=w518) -> ()  [unwired: 2 in, 3 out]
                                }
                              }
                            }
                          }
                        }
                      }
                      n224 = call "interpret Intensity.vi"("Intensity"=w464) -> ("Color"=w469:u32)  [unwired: 1 in, 1 out]
                      n225 = property on="Reference Intensity" class="Slide (strict)"("Fill Color"=w469) -> ()  [unwired: 2 in, 2 out]
                      n226 = local write "Reference Intensity"(w464) -> ()
                    }
                  }
                  frame #3 {
                    w529 = u8 0 ("Deaktiviert")
                    w526 = u8 0
                    n227 = Tick Count (ms)() -> (millisecond timer value=w530:u32)
                    n228 = control-ref of="3D Surface"() -> (w521:refnum<vi>)
                    n229 = call "stop Measurement.vi"("OCTDevice"=w533) -> ("OCTDevice"=w532:refnum<class "OCT Device.lvclass">)  [unwired: 5 in, 1 out]
                    n230 = call "clear Data.vi"("Data"=w527) -> ()  [unwired: 6 in, 1 out]
                    n231 = call "determine Surface.vi"("Surface Data in"=w525, "Data in"=w524) -> ("error out"=w522:errorcluster, "Surface Data out"=w523:refnum<class "Data.lvclass">)  [unwired: 3 in, 1 out]
                    "Surface" <- w523
                    n232 = call "Benchmark.vi"("TimeStart"=w531, "NumberOfBScans"=w536, "TimeFinish"=w530) -> ("FrameRate"=→"FrameRate":sgl)  [unwired: 1 in, 2 out]
                    n233 = call <vilib>:"Simple Error Handler.vi"("error in (no error)"=w528) -> ()  [unwired: 4 in, 5 out]
                    n234 = call <vilib>:"Unset Busy.vi"() -> ()  [unwired: 11 in, 1 out]
                    n235 = call-poly "display Data.vi"("error in (no error)"=w522, "Data in"=w523, "3D Surface Refnum"=w521) -> ()  [unwired: 2 in, 3 out]
                    n236 = property on="Measure" class="Bool"("Disabled"=w526) -> ()  [unwired: 2 in, 2 out]
                    n237 = property on="Recalibrate" class="Bool"("Disabled"=w526) -> ()  [unwired: 2 in, 2 out]
                    n238 = property on="Save" class="Bool"("Disabled"=w526) -> ()  [unwired: 2 in, 2 out]
                    n239 = property on="Number Scans X" class="DigNum (strict)"("Disabled"=w526) -> ()  [unwired: 2 in, 2 out]
                    n240 = property on="Number Scans Y" class="DigNum (strict)"("Disabled"=w526) -> ()  [unwired: 2 in, 2 out]
                    n241 = property on="Range X [mm]" class="DigNum (strict)"("Disabled"=w526) -> ()  [unwired: 2 in, 2 out]
                    n242 = property on="Range Y [mm]" class="DigNum (strict)"("Disabled"=w526) -> ()  [unwired: 2 in, 2 out]
                    n243 = property on="Level Surface" class="Bool (strict)"("Disabled"=w526) -> ()  [unwired: 2 in, 2 out]
                    n244 = property on="Petzval Filter" class="Bool (strict)"("Disabled"=w526) -> ()  [unwired: 2 in, 2 out]
                    n245 = property on="Median Filter" class="Bool (strict)"("Disabled"=w526) -> ()  [unwired: 2 in, 2 out]
                    n246 = property on="SizeFilter" class="DigNum (strict)"("Disabled"=w526) -> ()  [unwired: 2 in, 2 out]
                    n247 = property on="X" class="Slide (strict)"("Disabled"=w529) -> ()  [unwired: 2 in, 2 out]
                    n248 = property on="Y" class="Slide (strict)"("Disabled"=w529) -> ()  [unwired: 2 in, 2 out]
                    n249 = property on="Z" class="Slide (strict)"("Disabled"=w529) -> ()  [unwired: 2 in, 2 out]
                    n250 = property on="QuitApp" class="Bool (strict)"("Disabled"=w526) -> ()  [unwired: 2 in, 2 out]
                    "Volume" <- w524
                  }
                }
                n251 = local write "Progress"(w370) -> ()
                n252 = property on="Progress" class="Slide (strict)"("Visible"=w369) -> ()  [unwired: 2 in, 2 out]
              }
            }
          }
          event "Test Mode": Value Change {
            n253 = event-data() -> ()  [unwired: 1 in, 1 out]
            n254 = case shown="True" "Test Mode" {
              tunnel: w542 -> [w543 w558]
              tunnel: [w543 w556] -> w540
              tunnel: w538 -> [_ w552]
              tunnel: w539 -> [_ w551]
              frame False {
              }
              frame True {
                n255 = flat-sequence {
                  tunnel: [w574] -> w561
                  tunnel: [w586] -> w559
                  tunnel: w558 -> [w585]
                  tunnel: [w582] -> w555
                  tunnel: [w578] -> w553
                  tunnel: w552 -> [w578]
                  tunnel: [w579] -> _
                  tunnel: w551 -> [w579]
                  tunnel: [w573] -> w549
                  tunnel: [w572] -> w548
                  tunnel: [w565] -> w545
                  tunnel: [w564] -> w544
                  tunnel: w559 -> [w603]
                  tunnel: [w602] -> w562
                  tunnel: w561 -> [w601]
                  tunnel: [w600] -> w560
                  tunnel: [w599] -> w557
                  tunnel: w555 -> [w598]
                  tunnel: [w598] -> w554
                  tunnel: w553 -> [w597]
                  tunnel: [w596] -> w550
                  tunnel: w549 -> [w595]
                  tunnel: w548 -> [w594]
                  tunnel: [w593] -> w547
                  tunnel: [w592] -> w546
                  tunnel: w545 -> [w591]
                  tunnel: w544 -> [w590]
                  tunnel: w562 -> [w645]
                  tunnel: w560 -> [w650]
                  tunnel: w557 -> [w648]
                  tunnel: [w649] -> w556
                  tunnel: w554 -> [w647]
                  tunnel: w550 -> [w646]
                  tunnel: w547 -> [w644]
                  tunnel: w546 -> [w643]
                  frame #0 {
                    w571 = T13."Disabled and Grayed Out" ("Disabled")
                    n256 = property on="X" class="Slide (strict)"() -> (error out=w583:errorcluster, "Disabled"=w582:u8)  [unwired: 2 in, 1 out]
                    n257 = local read "Number Scans X"() -> (w580:i32)
                    n258 = local read "Range X [mm]"() -> (w581:dbl)
                    n259 = local write "Tab Control"(enum32{"B-Scan", "Surface"}."B-Scan" ("Tab Control")) -> ()
                    n260 = property on="Averaging*Binning" class="Slide (strict)"("Disabled"=w571) -> ()  [unwired: 2 in, 2 out]
                    n261 = property on="Averaging-Binning-Ratio" class="Slide (strict)"("Disabled"=w571) -> ()  [unwired: 2 in, 2 out]
                    n262 = property on="X" class="Slide (strict)"(error in=w583, "Disabled"=w571) -> ()  [unwired: 1 in, 2 out]
                    n263 = property on="Y" class="Slide (strict)"("Disabled"=w571) -> ()  [unwired: 2 in, 2 out]
                    n264 = property on="Z" class="Slide (strict)"("Disabled"=w571) -> ()  [unwired: 2 in, 2 out]
                    n265 = property on="OnlineDisplay" class="Bool (strict)"("Disabled"=w571) -> ()  [unwired: 2 in, 2 out]
                    n266 = property on="Measure" class="Bool"("Disabled"=w571) -> ()  [unwired: 2 in, 2 out]
                    n267 = property on="Frame" class="IntGraph (strict)"("XScale.NameLbl.Text"="Width (X) [mm]" ("X Scale.Name Label.Text"), "YScale.NameLbl.Text"="Depth (Z) [mm]" ("Y Scale.Name Label.Text")) -> ()  [unwired: 2 in, 2 out]
                    n268 = call "create B-Scan Pattern.vi"("AScans"=w580, "Range"=w581, "Probe"=w579) -> ("error out"=w563:errorcluster, "Scan Pattern"=w577:refnum<class "Scan Pattern.lvclass">, "Probe"=w564:refnum<class "Probe.lvclass">)  [unwired: 3 in]
                    n269 = local read "Angle [rad]"() -> (w576:dbl)
                    n270 = local read "Shift X [mm]"() -> (w567:dbl)
                    n271 = local read "Shift Y [mm]"() -> (w566:dbl)
                    n272 = property on="Recalibrate" class="Bool"("Disabled"=w571) -> ()  [unwired: 2 in, 2 out]
                    n273 = property on="Level Surface" class="Bool (strict)"("Disabled"=w571) -> ()  [unwired: 2 in, 2 out]
                    n274 = property on="Petzval Filter" class="Bool (strict)"("Disabled"=w571) -> ()  [unwired: 2 in, 2 out]
                    n275 = property on="Median Filter" class="Bool (strict)"("Disabled"=w571) -> ()  [unwired: 2 in, 2 out]
                    n276 = property on="SizeFilter" class="DigNum (strict)"("Disabled"=w571) -> ()  [unwired: 2 in, 2 out]
                    n277 = property on="Save" class="Bool"("Disabled"=w571) -> ()  [unwired: 2 in, 2 out]
                    n278 = call "rotate Scan Pattern.vi"("error in (no error)"=w563, "Angle"=w576, "ScanPattern"=w577) -> ("error out"=w568:errorcluster, "ScanPattern"=w570:refnum<class "Scan Pattern.lvclass">)  [unwired: 3 in]
                    n279 = call "shift Scan Pattern.vi"("error in (no error)"=w568, "Shift Y"=w566, "Shift X"=w567, "Scan Pattern in"=w570) -> ("Scan Pattern out"=w569:refnum<class "Scan Pattern.lvclass">)  [unwired: 2 in, 1 out]
                    n280 = property on="Number Scans Y" class="DigNum (strict)"("Disabled"=w571) -> ()  [unwired: 2 in, 2 out]
                    n281 = property on="Range Y [mm]" class="DigNum (strict)"("Disabled"=w571) -> ()  [unwired: 2 in, 2 out]
                    n282 = property on="Range X [mm]" class="DigNum (strict)"("Disabled"=w571) -> ()  [unwired: 2 in, 2 out]
                    n283 = property on="Number Scans X" class="DigNum (strict)"("Disabled"=w571) -> ()  [unwired: 2 in, 2 out]
                    n284 = call "check for Standby.vi"("ResetTimer"=TRUE) -> ()  [unwired: 2 out]
                    n285 = call "start Measurement.vi"("error in (no error)"=w563, "Acquisition Type"=T11."Asynchronous Continuous", "Scan Pattern"=w569, "OCTDevice"=w585) -> ("error out"=w586:errorcluster, "Scan Pattern"=w565:refnum<class "Scan Pattern.lvclass">, "OCTDevice"=w574:refnum<class "OCT Device.lvclass">)  [unwired: 1 in]
                    n286 = call "create Raw Data.vi"() -> ("Raw Data"=w572:refnum<class "Raw Data.lvclass">)  [unwired: 6 in, 1 out]
                    n287 = call "create Data.vi"() -> ("Data"=w573:refnum<class "Data.lvclass">)  [unwired: 6 in, 1 out]
                  }
                  frame #1 {
                    n288 = while {
                      tunnel: w601 -> [w630]
                      tunnel: [w635] -> w600
                      tunnel: [w607] -> w599
                      tunnel: w597 -> [w628]
                      shift-right: [w612] -> w602
                      shift-left: w603 -> [w618]
                      tunnel: [w631] -> w596
                      tunnel: w595 -> [w627]
                      tunnel: w594 -> [w629]
                      tunnel: [w616] -> w593
                      tunnel: [w615] -> w592
                      tunnel: w591 -> [w609]
                      tunnel: w590 -> [w606]
                      stop <- w631 continue-if-true
                      # "Will always be \"no error\",\nbut forces order of execution."
                      n289 = call "get Raw Data.vi"("error in (no error)"=w618, "Camera Index"=0, "RawData in"=w629, "OCTDevice in"=w630) -> ("error out"=w619:errorcluster, "RawData out"=w625:refnum<class "Raw Data.lvclass">, "OCTDevice out"=w607:refnum<class "OCT Device.lvclass">)  [unwired: 1 in]
                      n290 = call-poly "set Processing Output.vi"("error in (no error)"=w618, "Data"=w627, "Processing"=w628) -> ("error out"=w624:errorcluster, "Data"=w623:refnum<class "Data.lvclass">, "Processing"=w626:refnum<class "Processing.lvclass">)  [unwired: 2 in]
                      n291 = local read "Colored Data"() -> (w613:refnum<class "Colored Data.lvclass">)
                      n292 = control-ref of="Frame"() -> (w621:refnum<vi>)
                      n293 = call "execute Processing.vi"("error in (no error)"=w624, "Raw Data"=w625, "Processing"=w626) -> ("error out"=w622:errorcluster, "Raw Data"=w615:refnum<class "Raw Data.lvclass">, "Processing"=w617:refnum<class "Processing.lvclass">)  [unwired: 2 in]
                      n294 = call-poly "display Data.vi"("error in (no error)"=w622, "Data in"=w623, "IntGraph Refnum"=w621) -> ("error out"=w620:errorcluster, "Data out"=w616:refnum<class "Data.lvclass">)  [unwired: 2 in, 1 out]
                      n295 = call "get Relative Reference Intensity.vi"("Processing"=w617, "OCTDevice"=w607) -> ("Relative Reference Intensity"=w614:dbl)  [unwired: 2 in, 3 out]
                      "Reference Intensity" <- w614
                      n296 = local read "Test Mode"() -> (w639:bool)
                      n297 = local read "QuitApp"() -> (w638:bool)
                      n298 = call "interpret Intensity.vi"("Intensity"=w614) -> ("Color"=w634:u32)  [unwired: 1 in, 1 out]
                      n299 = Merge Errors(w620, w619) -> (w611:errorcluster)
                      n300 = call "get Camera Image.vi"("error in (no error)"=w611, "Colored Data in"=w613, "OCTDevice in"=w607) -> ("error out"=w608:errorcluster)  [unwired: 4 in, 2 out]
                      n301 = call "visualize Scan Pattern.vi"("error in (no error)"=w608, "Scan Pattern in"=w609, "Probe"=w606, "OCT Device"=w607) -> ("error out"=w605:errorcluster)  [unwired: 1 in, 3 out]
                      n302 = call "check for Standby.vi"() -> ("TimeOut"=w635:bool)  [unwired: 1 in, 1 out]
                      n303 = Not(x=w638) -> (.not. x?=w637:bool)
                      n304 = property on="Reference Intensity" class="Slide (strict)"("Fill Color"=w634) -> ()  [unwired: 2 in, 2 out]
                      n305 = Unbundle By Name(w611) -> ("status"=w633:bool)
                      n306 = Not(x=w635) -> (.not. x?=w636:bool)
                      n307 = Not(x=w633) -> (.not. x?=w632:bool)
                      n308 = Compound Arithmetic op=AND(w639, w637, w636, w632) -> (w631:bool)
                      n309 = call <vilib>:"Clear Errors.vi"("error in (no error)"=w605) -> ("error out"=w610:errorcluster)  [unwired: 6 in]
                      n310 = Merge Errors(w611, w610) -> (w612:errorcluster)
                    }
                  }
                  frame #2 {
                    w640 = T13."Enabled" ("Disabled")
                    n311 = call "clear Data.vi"("Data"=w644) -> ()  [unwired: 6 in, 1 out]
                    n312 = call "clear Raw Data.vi"("Raw Data"=w643) -> ()  [unwired: 6 in, 1 out]
                    n313 = local write "Test Mode Indicator"(w646) -> ()
                    n314 = call <vilib>:"Simple Error Handler.vi"("error in (no error)"=w645) -> ()  [unwired: 4 in, 5 out]
                    n315 = local write "Test Mode"(w646) -> ()
                    n316 = local read "Volume"() -> (w642:refnum<class "Data.lvclass">)
                    n317 = property on="X" class="Slide (strict)"("Disabled"=w647) -> ()  [unwired: 2 in, 2 out]
                    n318 = property on="Y" class="Slide (strict)"("Disabled"=w647) -> ()  [unwired: 2 in, 2 out]
                    n319 = property on="Z" class="Slide (strict)"("Disabled"=w647) -> ()  [unwired: 2 in, 2 out]
                    n320 = property on="Measure" class="Bool"("Disabled"=w640) -> ()  [unwired: 2 in, 2 out]
                    n321 = property on="OnlineDisplay" class="Bool (strict)"("Disabled"=w640) -> ()  [unwired: 2 in, 2 out]
                    n322 = property on="Recalibrate" class="Bool"("Disabled"=w640) -> ()  [unwired: 2 in, 2 out]
                    n323 = property on="Number Scans X" class="DigNum (strict)"("Disabled"=w640) -> ()  [unwired: 2 in, 2 out]
                    n324 = property on="Number Scans Y" class="DigNum (strict)"("Disabled"=w640) -> ()  [unwired: 2 in, 2 out]
                    n325 = property on="Range X [mm]" class="DigNum (strict)"("Disabled"=w640) -> ()  [unwired: 2 in, 2 out]
                    n326 = property on="Range Y [mm]" class="DigNum (strict)"("Disabled"=w640) -> ()  [unwired: 2 in, 2 out]
                    n327 = property on="Averaging*Binning" class="Slide (strict)"("Disabled"=w640) -> ()  [unwired: 2 in, 2 out]
                    n328 = property on="Averaging-Binning-Ratio" class="Slide (strict)"("Disabled"=w640) -> ()  [unwired: 2 in, 2 out]
                    n329 = call "is Data valid.vi"("Data"=w642) -> ("valid?"=w641:bool)
                    n330 = call "activate Standby.vi"("StandBy"=w650, "OCTDevice"=w648) -> ()  [unwired: 4 in, 2 out]
                    n331 = call "stop Measurement.vi"("OCTDevice"=w648) -> ("OCTDevice"=w649:refnum<class "OCT Device.lvclass">)  [unwired: 5 in, 1 out]
                    n332 = case shown="True" w641 {
                      frame False {
                      }
                      frame True {
                        n333 = property on="Save" class="Bool"("Disabled"=T13."Enabled") -> ()  [unwired: 2 in, 2 out]
                      }
                    }
                  }
                }
              }
            }
            "Test Mode Indicator" <- "Test Mode"
          }
          event "Tab Control": Value Change {
            n334 = event-data() -> ()  [unwired: 1 in, 6 out]
            n335 = local read "Tab Control"() -> (w652:enum32{"B-Scan", "Surface"})
            n336 = case shown="\"B-Scan\", Default" w652 {
              frame "B-Scan", Default {
                w654 = u8 2 ("Deaktiviert")
                w655 = u8 0 ("Deaktiviert")
                n337 = property on="X" class="Slide (strict)"("Disabled"=w655) -> ()  [unwired: 2 in, 2 out]
                n338 = property on="Y" class="Slide (strict)"("Disabled"=w655) -> ()  [unwired: 2 in, 2 out]
                n339 = property on="Z" class="Slide (strict)"("Disabled"=w655) -> ()  [unwired: 2 in, 2 out]
                n340 = property on="Level Surface" class="Bool (strict)"("Disabled"=w654) -> ()  [unwired: 2 in, 2 out]
                n341 = property on="Petzval Filter" class="Bool (strict)"("Disabled"=w654) -> ()  [unwired: 2 in, 2 out]
                n342 = property on="Median Filter" class="Bool (strict)"("Disabled"=w654) -> ()  [unwired: 2 in, 2 out]
                n343 = property on="SizeFilter" class="DigNum (strict)"("Disabled"=w654) -> ()  [unwired: 2 in, 2 out]
              }
              frame "Surface" {
                w657 = u8 0 ("Deaktiviert")
                w656 = u8 2 ("Deaktiviert")
                n344 = property on="X" class="Slide (strict)"("Disabled"=w656) -> ()  [unwired: 2 in, 2 out]
                n345 = property on="Y" class="Slide (strict)"("Disabled"=w656) -> ()  [unwired: 2 in, 2 out]
                n346 = property on="Z" class="Slide (strict)"("Disabled"=w656) -> ()  [unwired: 2 in, 2 out]
                n347 = property on="Level Surface" class="Bool (strict)"("Disabled"=w657) -> ()  [unwired: 2 in, 2 out]
                n348 = property on="Petzval Filter" class="Bool (strict)"("Disabled"=w657) -> ()  [unwired: 2 in, 2 out]
                n349 = property on="Median Filter" class="Bool (strict)"("Disabled"=w657) -> ()  [unwired: 2 in, 2 out]
                n350 = property on="SizeFilter" class="DigNum (strict)"("Disabled"=w657) -> ()  [unwired: 2 in, 2 out]
              }
            }
          }
          event "Range Y [mm]", "Number Scans Y", "Number Scans X", "Range X [mm]": Value Change {
            n351 = event-data() -> ()  [unwired: 1 in, 1 out]
            n352 = local read "Number Scans X"() -> (w663:i32)
            n353 = local read "Number Scans Y"() -> (w658:i32)
            n354 = Divide(x="Range X [mm]", y=w663) -> (x/y=w667:dbl)
            n355 = Divide(x="Range Y [mm]", y=w658) -> (x/y=w660:dbl)
            n356 = Multiply(x=1000.0, y=w667) -> (x*y=→"Spacing X [µm]":dbl)
            n357 = Multiply(x=1000.0, y=w660) -> (x*y=→"Spacing Y [µm]":dbl)
          }
          event "Recalibrate": Value Change {
            n358 = event-data() -> ()  [unwired: 1 in, 1 out]
            n359 = case shown="True" "Recalibrate" {
              tunnel: w670 -> [_ w674]
              tunnel: w669 -> [_ w673]
              frame False {
              }
              frame True {
                n360 = call "measure Calibration.vi"("Camera Index"=0, "Calibration Data"=Calibration_Selection."Offset Errors", "Processing"=w673, "OCTDevice"=w674) -> ()  [unwired: 2 in, 3 out]
              }
            }
          }
          event "X": Value Change {
            n361 = event-data() -> ()  [unwired: 1 in, 1 out]
            n362 = local read "Volume"() -> (w684:refnum<class "Data.lvclass">)
            n363 = call "create Data.vi"() -> ("error out"=w678:errorcluster, "Data"=w685:refnum<class "Data.lvclass">)  [unwired: 6 in]
            n364 = control-ref of="Frame"() -> (w680:refnum<vi>)
            n365 = property on="Frame" class="IntGraph (strict)"("x-Achse.Namensbeschriftung.Text"="Length (Y) [mm]" ("X Scale.Name Label.Text"), "y-Achse.Namensbeschriftung.Text"="Depth (Z) [mm]" ("Y Scale.Name Label.Text")) -> ()  [unwired: 2 in, 2 out]
            n366 = call "get Data Slice Pos.vi"("Normal Direction"=Normal_Direction_Selection."Direction 2", "error in (no error)"=w678, "Position"="X", "Slice"=w685, "Data"=w684) -> ("error out"=w677:errorcluster, "Slice"=w682:refnum<class "Data.lvclass">)  [unwired: 2 in, 1 out]
            n367 = call-poly "display Data.vi"("error in (no error)"=w677, "Data in"=w682, "IntGraph Refnum"=w680) -> ("error out"=w676:errorcluster, "Data out"=w679:refnum<class "Data.lvclass">)  [unwired: 2 in, 1 out]
            n368 = call "clear Data.vi"("error in (no error)"=w676, "Data"=w679) -> ()  [unwired: 5 in, 1 out]
          }
          event "Y": Value Change {
            n369 = event-data() -> ()  [unwired: 1 in, 6 out]
            n370 = call "create Data.vi"() -> ("error out"=w691:errorcluster, "Data"=w700:refnum<class "Data.lvclass">)  [unwired: 6 in]
            n371 = local read "Volume"() -> (w699:refnum<class "Data.lvclass">)
            n372 = control-ref of="Frame"() -> (w696:refnum<vi>)
            n373 = property on="Frame" class="IntGraph (strict)"("x-Achse.Namensbeschriftung.Text"="Width (X) [mm]" ("X Scale.Name Label.Text"), "y-Achse.Namensbeschriftung.Text"="Depth (Z) [mm]" ("Y Scale.Name Label.Text")) -> ()  [unwired: 2 in, 2 out]
            n374 = call "get Data Slice Pos.vi"("Normal Direction"=Normal_Direction_Selection."Direction 3", "error in (no error)"=w691, "Position"="Y", "Slice"=w700, "Data"=w699) -> ("error out"=w690:errorcluster, "Slice"=w697:refnum<class "Data.lvclass">)  [unwired: 2 in, 1 out]
            n375 = call-poly "display Data.vi"("error in (no error)"=w690, "Data in"=w697, "IntGraph Refnum"=w696) -> ("error out"=w689:errorcluster, "Data out"=w695:refnum<class "Data.lvclass">)  [unwired: 2 in, 1 out]
            n376 = call "clear Data.vi"("error in (no error)"=w689, "Data"=w695) -> ()  [unwired: 5 in, 1 out]
          }
          event "Z": Value Change {
            n377 = event-data() -> ()  [unwired: 1 in, 1 out]
            n378 = call "create Data.vi"() -> ("error out"=w704:errorcluster, "Data"=w713:refnum<class "Data.lvclass">)  [unwired: 6 in]
            n379 = local read "Volume"() -> (w712:refnum<class "Data.lvclass">)
            n380 = control-ref of="Frame"() -> (w709:refnum<vi>)
            n381 = call "get Data Slice Pos.vi"("Normal Direction"=Normal_Direction_Selection."Direction 1", "error in (no error)"=w704, "Position"="Z", "Slice"=w713, "Data"=w712) -> ("error out"=w703:errorcluster, "Slice"=w710:refnum<class "Data.lvclass">)  [unwired: 2 in, 1 out]
            n382 = property on="Frame" class="IntGraph (strict)"("x-Achse.Namensbeschriftung.Text"="Width (X) [mm]" ("X Scale.Name Label.Text"), "y-Achse.Namensbeschriftung.Text"="Length (Y) [mm]" ("Y Scale.Name Label.Text")) -> ()  [unwired: 2 in, 2 out]
            n383 = call-poly "display Data.vi"("error in (no error)"=w703, "Data in"=w710, "IntGraph Refnum"=w709) -> ("error out"=w702:errorcluster, "Data out"=w708:refnum<class "Data.lvclass">)  [unwired: 2 in, 1 out]
            n384 = call "clear Data.vi"("error in (no error)"=w702, "Data"=w708) -> ()  [unwired: 5 in, 1 out]
          }
        }
      }
      n385 = while {
        tunnel: w141 -> [w145]
        tunnel: w139 -> [w144]
        tunnel: w138 -> [w143]
        stop <- w146 stop-if-true
        n386 = event shown="[1] \"Options\": Value Change" {
          selector: _ -> [_ _ _ _ _ _ _ _ _ _]
          dyn-events: _ -> [_ _ _ _ _ _ _ _ _ _]
          timeout: 500 -> [_ _ _ _ _ _ _ _ _ _]
          tunnel: w145 -> [_ w150 _ _ _ w189 _ _ _ _]
          tunnel: w144 -> [_ w149 _ w164 _ _ _ _ w198 _]
          tunnel: w143 -> [_ w148 _ w165 _ _ _ _ _ _]
          event Timeout {
            n387 = event-data() -> ()  [unwired: 1 in, 2 out]
          }
          event "Options": Value Change {
            n388 = event-data() -> ()  [unwired: 1 in, 1 out]
            n389 = case shown="True" "Options" {
              tunnel: w149 -> [_ w157]
              tunnel: [FALSE ("Options") FALSE ("Options")] -> w152
              tunnel: w150 -> [_ w155]
              tunnel: w148 -> [_ w154]
              frame False {
              }
              frame True {
                n390 = call "Options Dialog.vi"("GalvoControl"=w154, "Processing"=w157, "OCT Device"=w155) -> ()  [unwired: 1 in]
              }
            }
            n391 = local write "Options"(w152) -> ()
          }
          event "Saturation", "Contrast", "Brightness": Value Change {
            n392 = event-data() -> ()  [unwired: 1 in, 1 out]
          }
          event "Averaging*Binning", "Averaging-Binning-Ratio", "Range X [mm]", "Number Scans X": Value Change {
            n393 = event-data() -> ()  [unwired: 1 in, 1 out]
            n394 = Decrement(x="Averaging*Binning") -> (x-1=w173:i32)
            n395 = Multiply(x=w173, y="Averaging-Binning-Ratio") -> (x*y=w170:dbl)
            n396 = To Long Integer(number=w170) -> (32bit integer=w171:i32)
            n397 = Increment(x=w173) -> (x+1=w172:i32)
            n398 = Increment(x=w171) -> (x+1=w167:i32)
            n399 = Quotient & Remainder(x=w172, y=w167) -> (floor(x/y)=w168:i32)  [unwired: 1 out]
            n400 = call "set Probe Parameter Int.vi"("Value"="Averaging*Binning", "Probe Parameter Int"=Probe_Parameter_Int_Selection."Oversampling", "GalvoControl"=w165) -> ("error out"=w160:errorcluster)  [unwired: 3 in, 1 out]
            n401 = call "set Processing Parameter Int.vi"("error in (no error)"=w160, "Value"=w168, "Processing Paramter Int Selection"=Processing_Parameter_Int_Selection."Spectrum Averaging", "Processing in"=w164) -> ("error out"=w161:errorcluster, "Processing out"=w159:refnum<class "Processing.lvclass">)  [unwired: 2 in]
            n402 = call "set Processing Parameter Int.vi"("error in (no error)"=w161, "Value"=w167, "Processing Paramter Int Selection"=Processing_Parameter_Int_Selection."A-Scan Averaging", "Processing in"=w159) -> ()  [unwired: 2 in, 2 out]
          }
          event "Boundries": Value Change {
            n403 = event-data() -> ()  [unwired: 1 in, 5 out]
            n404 = control-ref of="Frame"() -> (w176:refnum<vi>)
            n405 = local read "Coloring"() -> (w183:refnum<class "Coloring.lvclass">)
            n406 = call "clear Coloring.vi"("Coloring"=w183) -> ("error out"=w180:errorcluster)  [unwired: 6 in]
            n407 = call "Palette Graph.vi"("Reference to the B-scan Graph"=w176, "Boundaries"="Boundries", "Color Scheme"="Color Scheme") -> ()
            n408 = call "create Coloring.vi"("error in (no error)"=w180, "Color Byte Order"=Coloring_Byteorder."RGBA32", "Color Table Selection"="Color Scheme") -> ("error out"=w181:errorcluster, "Coloring"=w184:refnum<class "Coloring.lvclass">)  [unwired: 3 in]
            n409 = Unbundle("Boundries") -> (w179:sgl, w178:sgl)
            n410 = call "set Coloring Boundaries.vi"("error in (no error)"=w181, "Danymic Range High [dB]"=w178, "Dynamic Range Low [dB]"=w179, "Coloring in"=w184) -> ("error out"=w175:errorcluster, "Coloring out"=w182:refnum<class "Coloring.lvclass">)  [unwired: 2 in]
            n411 = local write "Coloring"(w182) -> ()
            n412 = call <vilib>:"Simple Error Handler.vi"("error in (no error)"=w175) -> ()  [unwired: 4 in, 5 out]
          }
          event "Light": Value Change {
            n413 = event-data() -> ()  [unwired: 1 in, 1 out]
            n414 = call "set Output Device Value by Name.vi"("Value"="Light", "Identifier"="ring light", "OCTDevice"=w189) -> ("error out"=w186:errorcluster)  [unwired: 3 in, 1 out]
            n415 = call <vilib>:"Simple Error Handler.vi"("error in (no error)"=w186) -> ()  [unwired: 4 in, 5 out]
          }
          event Mouse Down {
            n416 = event-data() -> ()  [unwired: 1 in, 5 out]
            n417 = call "check for Standby.vi"("ResetTimer"=TRUE) -> ()  [unwired: 2 out]
          }
          event "QuitApp": Mouse Enter {
            w191 = u32 16448250
            n418 = event-data() -> ()  [unwired: 1 in, 4 out]
            n419 = Bundle(u32 16711680, u32 16448250) -> (w194:cluster{u32, u32})  [unwired: 1 in]
            n420 = Bundle(u32 8978432, w191) -> (w193:cluster{u32, u32})  [unwired: 1 in]
            n421 = Build Array(w194, w193) -> (w192:cluster{u32, u32}[])
            n422 = property on="QuitApp" class="Bool (strict)"("Colors [4]"=w192, "BoolText.TextColor"=w191) -> ()  [unwired: 2 in, 2 out]
          }
          event "Window": Value Change {
            n423 = event-data() -> ()  [unwired: 1 in, 1 out]
            n424 = call "set Apodization Window.vi"("Window"="Window", "Processing"=w198) -> ()  [unwired: 4 in, 2 out]
          }
          event "QuitApp": Mouse Leave {
            w201 = u32 0
            n425 = event-data() -> ()  [unwired: 1 in, 1 out]
            n426 = Bundle(u32 9868950, w201) -> (w202:cluster{u32, u32})  [unwired: 1 in]
            n427 = Bundle(u32 12369084, u32 0) -> (w203:cluster{u32, u32})  [unwired: 1 in]
            n428 = Build Array(w203, w202) -> (w200:cluster{u32, u32}[])
            n429 = property on="QuitApp" class="Bool (strict)"("Colors [4]"=w200, "BoolText.TextColor"=w201) -> ()  [unwired: 2 in, 2 out]
          }
        }
        n430 = local read "QuitApp"() -> (w146:bool)
      }
    }
    frame #4 {
      n431 = local read "Filtered Surface"() -> (w717:refnum<class "Data.lvclass">)
      n432 = local read "Colored Data"() -> (w718:refnum<class "Colored Data.lvclass">)
      n433 = local read "Volume"() -> (w715:refnum<class "Data.lvclass">)
      n434 = local read "Surface"() -> (w716:refnum<class "Data.lvclass">)
      n435 = call "clear Data.vi"("Data"=w715) -> ()  [unwired: 6 in, 1 out]
      n436 = call "clear Data.vi"("Data"=w716) -> ()  [unwired: 6 in, 1 out]
      n437 = call "clear Colored Data.vi"("Colored Data"=w718) -> ()  [unwired: 6 in, 1 out]
      n438 = call "clear Data.vi"("Data"=w717) -> ()  [unwired: 6 in, 1 out]
    }
    frame #5 {
      n439 = call "close Device.vi"("OCTDevice"=w721) -> ()  [unwired: 6 in, 1 out]
      n440 = call "IMAQ Dispose"("All Images? (No)"=TRUE) -> ()  [unwired: 5 in, 1 out]
    }
    frame #6 {
      n441 = local read "AutoSafe"() -> (w722:bool)
      n442 = case shown="True" w722 {
        frame False {
        }
        frame True {
          n443 = local read "Number Scans X"() -> (w736:i32)
          n444 = local read "Number Scans Y"() -> (w734:i32)
          n445 = local read "Color Scheme"() -> (w723:T1)
          n446 = call "get Config Path.vi"() -> ("Path"=w724:path)  [unwired: 1 in, 1 out]
          n447 = local read "Range X [mm]"() -> (w735:dbl)
          n448 = local read "Range Y [mm]"() -> (w733:dbl)
          n449 = local read "Light"() -> (w726:i32)
          n450 = local read "Brightness"() -> (w731:sgl)
          n451 = local read "Saturation"() -> (w732:sgl)
          n452 = local read "Contrast"() -> (w730:sgl)
          n453 = local read "Window"() -> (w725:T4)
          n454 = Build Path(base path=w724, name or relative path=path "Settings.ini" ("Relative \"SpectralRadar.ini\" Path")) -> (appended path=w757:path)
          n455 = call "init Settings.vi"("Path to settings file"=w757) -> ("Settings"=w755:refnum<class "Settings.lvclass">)  [unwired: 5 in, 1 out]
          n456 = call "set Settings Entry Int.vi"("Value"=w736, "Node"="ColumnsX", "Settings"=w755) -> ("Settings"=w754:refnum<class "Settings.lvclass">)  [unwired: 3 in, 1 out]
          n457 = call "set Settings Entry Float.vi"("Value"=w735, "Node"="RangeX", "Settings"=w754) -> ("Settings"=w753:refnum<class "Settings.lvclass">)  [unwired: 3 in, 1 out]
          n458 = call "set Settings Entry Int.vi"("Value"=w734, "Node"="ColumnsY", "Settings"=w753) -> ("Settings"=w752:refnum<class "Settings.lvclass">)  [unwired: 3 in, 1 out]
          n459 = call "set Settings Entry Float.vi"("Value"=w733, "Node"="RangeY", "Settings"=w752) -> ("Settings"=w737:refnum<class "Settings.lvclass">)  [unwired: 3 in, 1 out]
          n460 = call "set Settings Entry Float.vi"("Value"=w732, "Node"="Saturation" ("Node Name"), "Settings"=w737) -> ("Settings"=w751:refnum<class "Settings.lvclass">)  [unwired: 3 in, 1 out]
          n461 = call "set Settings Entry Float.vi"("Value"=w731, "Node"="Brightness" ("Node Name"), "Settings"=w751) -> ("Settings"=w750:refnum<class "Settings.lvclass">)  [unwired: 3 in, 1 out]
          n462 = call "set Settings Entry Float.vi"("Value"=w730, "Node"="Contrast" ("Node Name"), "Settings"=w750) -> ("Settings"=w729:refnum<class "Settings.lvclass">)  [unwired: 3 in, 1 out]
          n463 = call "set Settings Entry Int.vi"("Value"=w726, "Node"="RingLight" ("Node Name"), "Settings"=w729) -> ("Settings"=w728:refnum<class "Settings.lvclass">)  [unwired: 3 in, 1 out]
          n464 = call "set Settings Entry Int.vi"("Value"=w725, "Node"="ApodizationWindow" ("Node Name"), "Settings"=w728) -> ("Settings"=w749:refnum<class "Settings.lvclass">)  [unwired: 3 in, 1 out]
          n465 = call "set Settings Entry Int.vi"("Value"=w723, "Node"="Palette" ("Node Name"), "Settings"=w749) -> ("Settings"=w748:refnum<class "Settings.lvclass">)  [unwired: 3 in, 1 out]
          n466 = call "save Settings.vi"("Settings"=w748) -> ("Settings"=w747:refnum<class "Settings.lvclass">)  [unwired: 5 in, 1 out]
          n467 = call "close Settings.vi"("Settings"=w747) -> ()  [unwired: 6 in, 1 out]
        }
      }
    }
  }
